vi "main_x.vi"() -> ()   [LabVIEW 2017]
uses:
  <vilib>/Instr/_visa.llb/VISA Configure Serial Port (Instr).vi
panel:
  in  "端口配置":bool
  in  "参数计算":bool
  in  "时漂测试间隔时间(min)":i32=1800000
  in  "时漂测试":bool
  out "时漂":dbl
  out "时漂测试数据":i32[](listbox)
  out "时漂常压输出":string[][](array[string])
  out "错误输出 3":errorcluster caption="错误输出"
  out "Yf.s":dbl[](array[numeric])
  in  "温度显示编号":enum16{""}(ring)
  out "曲线拟合参数":string
  in  "传感器显示编号":enum16{""}(ring)
  out "显示数据":i32[](listbox)
  out "XY图":cluster{dbl[], dbl[]}[](graph)
  out "结束":bool
  out "R5-1":dbl
  out "理论K":dbl
  out "RX":dbl[](array[numeric])
  out "电流":dbl
  out "放大倍数":dbl
  in  "Rx计算":bool
  in  "RsRb计算":bool
  out "Rp":dbl
  out "Rs":dbl
  out "显示数据":string[][](array[string])
  out "数据":string[][](array[string])
  out "错误输出 2":errorcluster caption="错误输出"
  out "压力稳定":bool
  out "压力最小值":dbl
  out "压力最大值":dbl
  out "保存名":string
  out "数据保存路径":path
  out "错误输出":errorcluster
  out "恒温结束时间":string
  out "恒温开始时间":string
  out "恒温结束分钟":i32
  out "恒温结束小时":i32
  out "分钟":i32
  out "小时":i32
  out "开始上电":bool
  out "恒温开始":bool
  out "开始采集":bool
  out "传感器预热":bool
  out "恒温中":bool
  out "温度校验次数":dbl
  out "实时压力kPa":string
  out "实时温度℃":dbl
  out "当前设定温度℃":dbl
  out "温度点":i32
  in  "温度（℃）":dbl[](array[numeric])
  in  "CONST820":refnum<visa-resource-name>="COM3"
  in  "传感器顺序编号（从1开始）":string[](array[string])
  in  "第二路电流 （A）":dbl=1.0
  in  "第二路电压（V）":dbl=5.0
  in  "第一路电压（V）":dbl=5.0
  in  "第一路电流（A）":dbl=1.0
  in  "DH1766-2":refnum<visa-resource-name>="COM5"
  in  "检定次数":i32=1
  in  "恒温时间（分钟）":i32
  in  "传感器预热时间（分钟）":i32
  in  "GWS":refnum<visa-resource-name>="COM4"
  in  "温度上限（℃）":dbl=75.0
  in  "温度下限（℃）":dbl=-45.0
  in  "HP34401":refnum<visa-resource-name>="COM1"
  in  "压力设定值（KPa）":dbl[](array[numeric])
  in  "STOP":bool
  out "loging":string
  out "HP34401A":bool caption="34401A"
  out "GWS":bool
  out "DH1766-2":bool
  out "CONST820":bool
  in  "START":bool
  # "多通道传感器测试系统"
  # "温度设置：如需要进行自动 参数计算，请设置20℃附近常温。如不需要请忽略。\n选择时漂测试 测试完成后会自动进行行程测试。单独点击开始 仅进行行程测试。\n传感器编号从1开始，逐加。\n如需进行时漂测试，请只设置常温常压。"
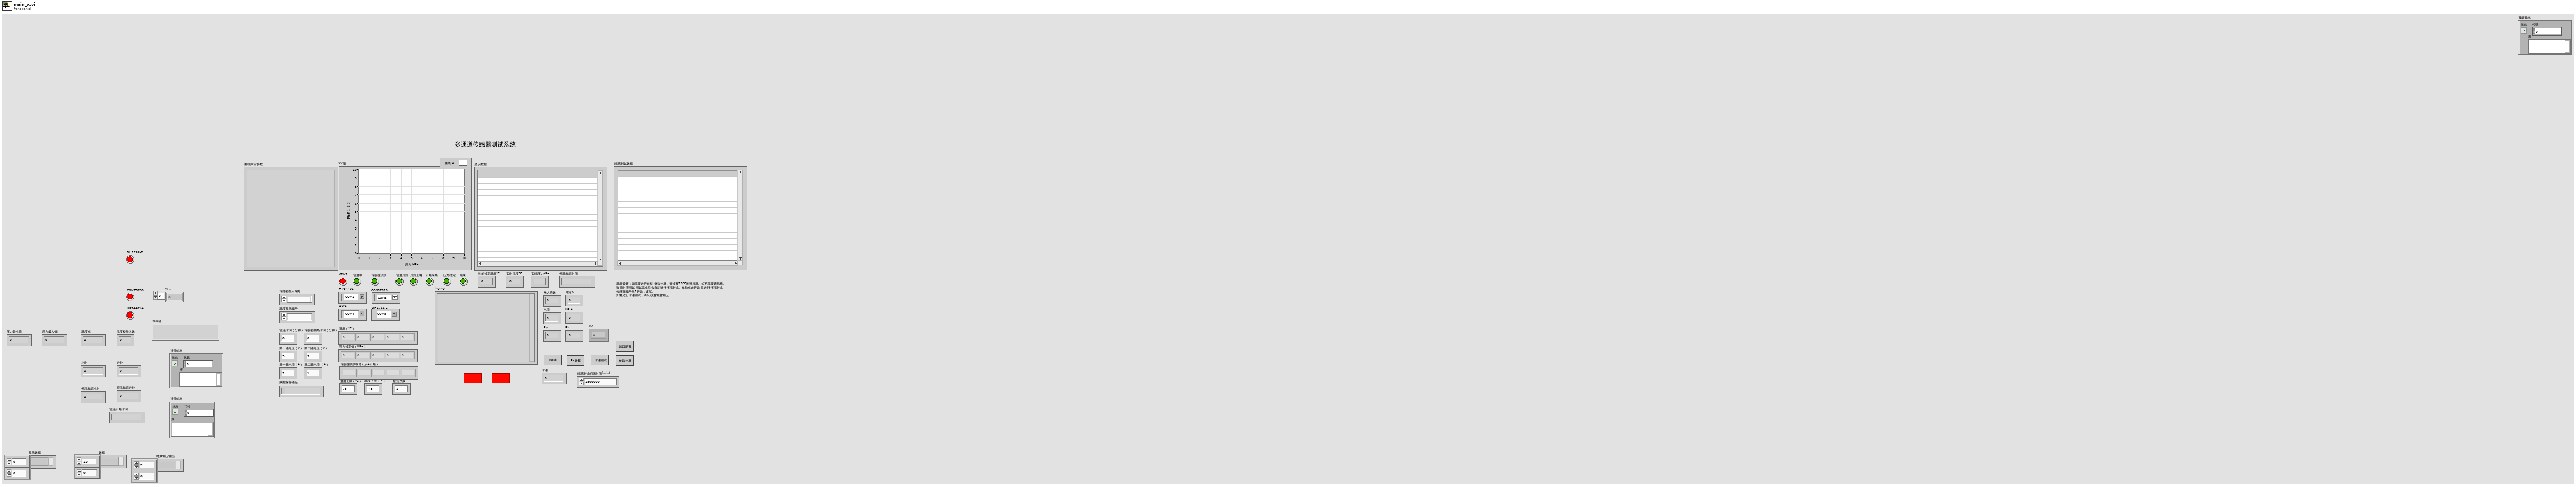
[diagram p1: front panel]
types:
  T1 = enum32{"Invalid", "Standard", "Closed", "Hidden", "Minimized", "Maximized"}
  T2 = enum8{"Enabled", "Disabled", "Disabled and Grayed Out"}
  T3 = enum16{"open", "open or create", "create or replace", "create", "open (read-only)"}
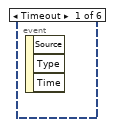
[diagram p2: hidden frame]
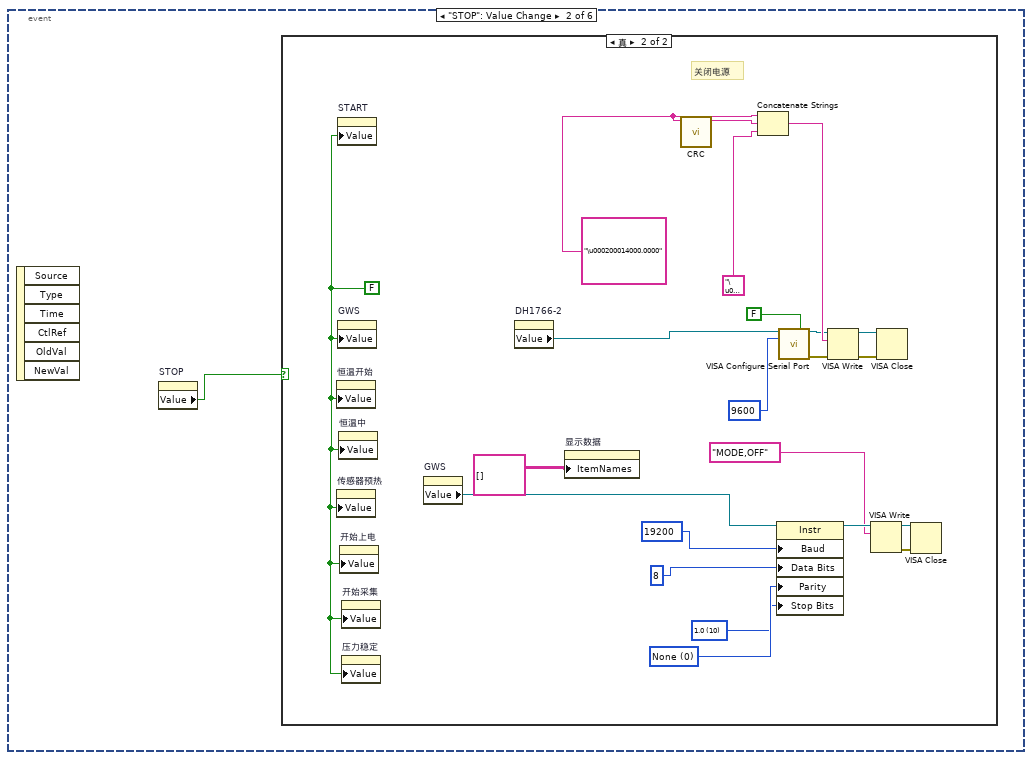
[diagram p3: hidden frame]
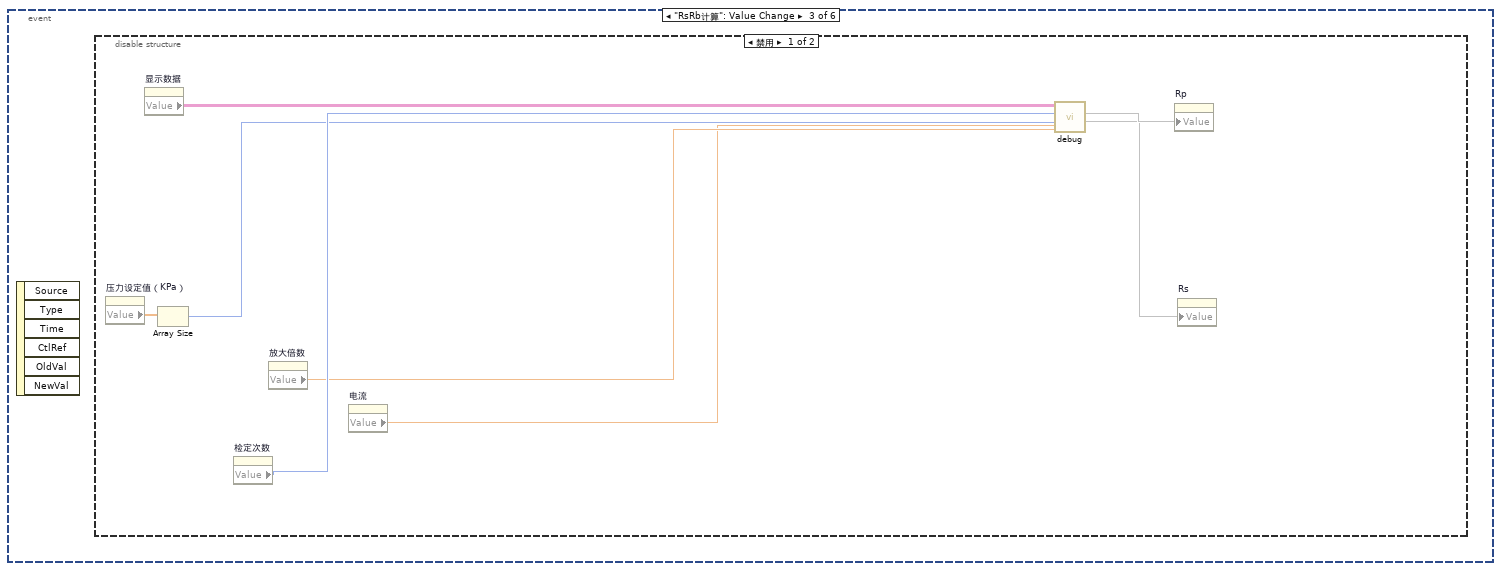
[diagram p5: hidden frame]
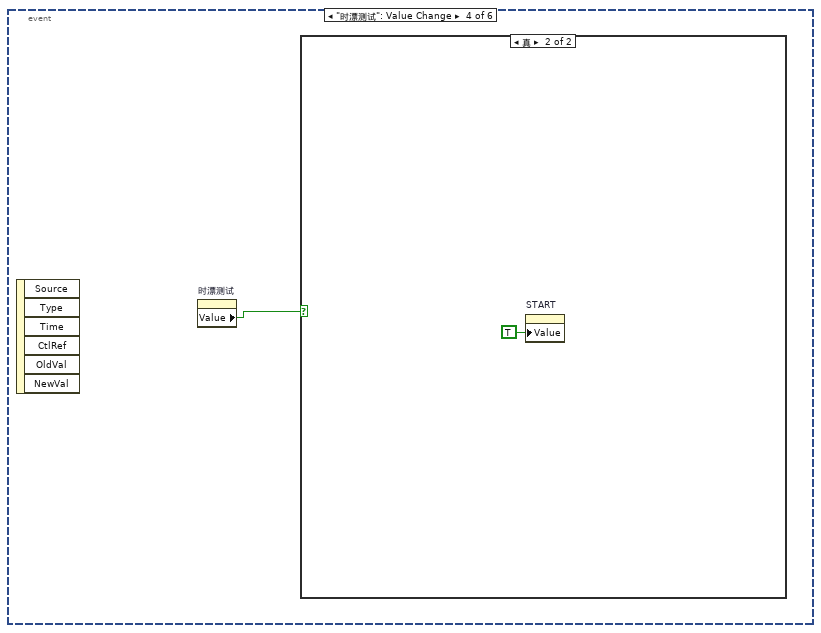
[diagram p7: hidden frame]
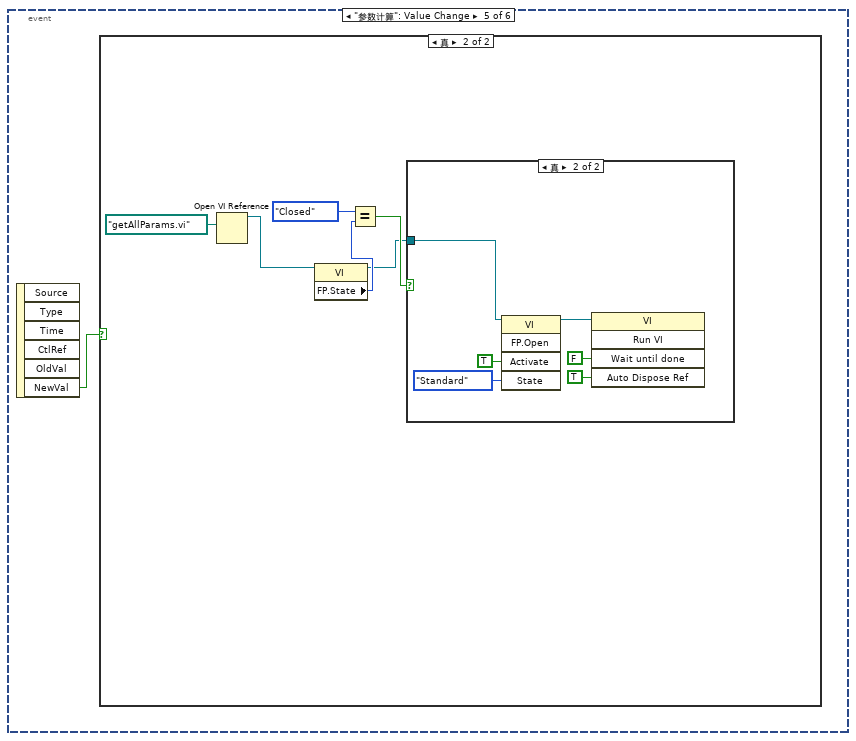
[diagram p9: hidden frame]
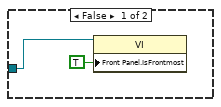
[diagram p11: hidden frame]
diagram:
  n1 = while {
    stop <- FALSE stop-if-true
    n2 = event shown="[5] \"Rx计算\": 值改变" {
      selector: _ -> [_ _ _ _ _ _]
      dyn-events: _ -> [_ _ _ _ _ _]
      timeout: _ -> [_ _ _ _ _ _]
      event Timeout {
        n3 = event-data() -> ()  [unwired: 1 in, 3 out]
      }
      event "STOP": Value Change {
        n4 = event-data() -> ()  [unwired: 1 in, 6 out]
        n5 = property on="STOP" class="Bool (严格)"() -> ("Value"=w2:bool)  [unwired: 2 in, 2 out]
        n6 = case shown="真" w2 {
          frame False {
          }
          frame True {
            w10 = u16 10 items=["1.0"=10, "1.5"=15, "2.0"=20] ("Serial Settings:Stop Bits")
            w11 = u16 0 items=["None", "Odd", "Even", "Mark", "Space"] ("Serial Settings:Parity")
            w9 = "\u000200014000.0000"
            w24 = FALSE ("START")
            # "关闭电源"
            n7 = property on="恒温开始" class="Bool (严格)"("Value"=w24) -> ()  [unwired: 2 in, 2 out]
            n8 = property on="传感器预热" class="Bool (严格)"("Value"=w24) -> ()  [unwired: 2 in, 2 out]
            n9 = property on="START" class="Bool (严格)"("Value"=w24) -> ()  [unwired: 2 in, 2 out]
            n10 = property on="GWS" class="Bool (严格)"("Value"=w24) -> ()  [unwired: 2 in, 2 out]
            n11 = property on="恒温中" class="Bool (严格)"("Value"=w24) -> ()  [unwired: 2 in, 2 out]
            n12 = property on="开始上电" class="Bool (严格)"("Value"=w24) -> ()  [unwired: 2 in, 2 out]
            n13 = property on="开始采集" class="Bool (严格)"("Value"=w24) -> ()  [unwired: 2 in, 2 out]
            n14 = property on="压力稳定" class="Bool (严格)"("Value"=w24) -> ()  [unwired: 2 in, 2 out]
            n15 = property on="GWS" class="VISAName"() -> ("Value"=w5:refnum<visa-resource-name>)  [unwired: 2 in, 2 out]
            n16 = property on="DH1766-2" class="VISAName"() -> ("Value"=w4:refnum<visa-resource-name>)  [unwired: 2 in, 2 out]
            n17 = property on="显示数据" class="MCListbox (严格)"("ItemNames"=string[][] []) -> ()  [unwired: 2 in, 2 out]
            n18 = call "CRC.vi"("命令字符串"=w9) -> ("校验字符串"=w23:string)  [unwired: 10 in]
            n19 = Concatenate Strings(w9, w23, "\u0003" ("字符串")) -> (w20:string)
            n20 = property class="Instr"(reference=w5, "Baud"=u32 19200 ("Serial Settings:Baud Rate"), "Data Bits"=u16 8 ("Serial Settings:Data Bits"), "Parity"=w11, "Stop Bits"=w10) -> (reference out=w17:refnum<visa-resource-name>)  [unwired: 1 in, 1 out]
            n21 = call-poly "VISA Configure Serial Port"("VISA resource name"=w4, "Enable Termination\nChar (T)"=FALSE ("Enable Termination\nChar (T)"), "baud rate (9600)"=u32 9600) -> ("VISA resource name out"=w19:refnum<visa-resource-name>, "error out"=w18:errorcluster)  [unwired: 4 in, 7 out]
            n22 = VISA Write(VISA resource name=w19, write buffer=w20, error in (no error)=w18) -> (VISA resource name out=w22:refnum<visa-resource-name>, error out=w21:errorcluster)  [unwired: 1 out]
            n23 = VISA Write(VISA resource name=w17, write buffer="MODE,OFF" ("写入缓冲区")) -> (VISA resource name out=w15:refnum<visa-resource-name>, error out=w16:errorcluster)  [unwired: 1 in, 1 out]
            n24 = VISA Close(VISA resource name=w22, error in (no error)=w21) -> ()  [unwired: 1 out]
            n25 = VISA Close(VISA resource name=w15, error in (no error)=w16) -> ()  [unwired: 1 out]
          }
        }
      }
      event "RsRb计算": Value Change {
        n26 = event-data() -> ()  [unwired: 1 in, 6 out]
        n27 = disable-structure shown="禁用" {
          frame Disabled {
            n28 = property on="压力设定值（KPa）" class="Arr (严格)"() -> ("Value"=w32:dbl[])  [unwired: 2 in, 2 out]
            n29 = property on="显示数据" class="Arr (严格)"() -> ("Value"=w31:string[][])  [unwired: 2 in, 2 out]
            n30 = Array Size(array=w32) -> (size(s)=w29:i32)
            n31 = property on="检定次数" class="DigNum (严格)"() -> ("Value"=w30:i32)  [unwired: 2 in, 2 out]
            n32 = property on="放大倍数" class="DigNum (严格)"() -> ("Value"=w28:dbl)  [unwired: 2 in, 2 out]
            n33 = property on="电流" class="DigNum (严格)"() -> ("Value"=w27:dbl)  [unwired: 2 in, 2 out]
            n34 = call "debug.vi"("I"=w27, "A"=w28, "压力点个数"=w29, "检定次数"=w30, 11:w31) -> (1:w25, 2:w26)  [unwired: 5 in]
            n35 = property on="Rp" class="DigNum (严格)"("Value"=w26) -> ()  [unwired: 2 in, 2 out]
            n36 = property on="Rs" class="DigNum (严格)"("Value"=w25) -> ()  [unwired: 2 in, 2 out]
          }
          frame Enabled {
          }
        }
      }
      event "时漂测试": Value Change {
        n37 = event-data() -> ()  [unwired: 1 in, 6 out]
        n38 = property on="时漂测试" class="Bool (严格)"() -> ("Value"=w33:bool)  [unwired: 2 in, 2 out]
        n39 = case shown="真" w33 {
          frame False {
          }
          frame True {
            n40 = property on="START" class="Bool (严格)"("Value"=TRUE ("START")) -> ()  [unwired: 2 in, 2 out]
          }
        }
      }
      event "参数计算": Value Change {
        n41 = event-data() -> ("NewVal"=w35:bool)  [unwired: 1 in, 5 out]
        n42 = case shown="真" w35 {
          frame False {
          }
          frame True {
            n43 = Open VI Reference(vi path=path "getAllParams.vi" ("VI路径")) -> (vi reference=w36:refnum<vi>)  [unwired: 5 in, 1 out]
            n44 = property class="VI"(reference=w36) -> (reference out=w37:refnum<vi>, "FP.State"=w40:T1)  [unwired: 1 in, 1 out]
            n45 = Equal?(x=T1."Closed", y=w40) -> (x = y?=w38:bool)
            n46 = case shown="真" w38 {
              tunnel: w37 -> [w42 w44]
              frame False {
                n47 = property class="VI"(reference=w42, "Front Panel.IsFrontmost"=TRUE ("前面板窗口:在最前")) -> ()  [unwired: 1 in, 2 out]
              }
              frame True {
                n48 = invoke class="VI" method="FP.Open"(reference=w44, "Activate"=TRUE ("激活？"), "State"=T1."Standard" ("状态")) -> (reference out=w47:refnum<vi>)  [unwired: 2 in, 4 out]
                n49 = invoke class="VI" method="Run VI"(reference=w47, "Wait until done"=FALSE ("结束前等待"), "Auto Dispose Ref"=TRUE ("自动销毁引用")) -> ()  [unwired: 2 in, 5 out]
              }
            }
          }
        }
      }
      event "Rx计算": Value Change {
        n50 = event-data() -> ()  [unwired: 1 in, 6 out]
        n51 = disable-structure shown="禁用" {
          frame Disabled {
            n52 = property on="压力设定值（KPa）" class="Arr (严格)" props=["Value"]() -> ()  [unwired: 2 in, 3 out]
            n53 = property on="数据" class="Arr (严格)" props=["Value"]() -> ()  [unwired: 2 in, 3 out]
            n54 = property on="压力设定值（KPa）" class="Arr (严格)"() -> ("Value"=w57:dbl[])  [unwired: 2 in, 2 out]
            n55 = Array Size(array=w57) -> (size(s)=w54:i32)
            n56 = property on="数据" class="Arr (严格)"() -> ("Value"=w56:string[][])  [unwired: 2 in, 2 out]
            n57 = property on="检定次数" class="DigNum (严格)"() -> ("Value"=w55:i32)  [unwired: 2 in, 2 out]
            n58 = property on="R5-1" class="DigNum (严格)"() -> ("Value"=w52:dbl)  [unwired: 2 in, 2 out]
            n59 = property on="理论K" class="DigNum (严格)"() -> ("Value"=w51:dbl)  [unwired: 2 in, 2 out]
            n60 = call "getCluster.vi"("数据"=w56, "检定次数"=w55, "压力点个数"=w54, "传感器索引（1开始）"=1, "R5-1"=w52, "理论 K"=w51) -> ("Rx"=w50:dbl[])  [unwired: 2 in, 7 out]
            n61 = property on="RX" class="Arr (严格)"("Value"=w50) -> ()  [unwired: 2 in, 2 out]
          }
          frame Enabled {
          }
        }
      }
    }
  }
  n62 = flat-sequence {
    frame #0 {
      w59 = string[][] []
      w65 = ""
      w66 = 0.0
      w63 = FALSE
      # "时漂测试开始不用规定"
      n63 = disable-structure shown="禁用" {
        frame Disabled {
          n64 = property on="检定次数" class="DigNum (严格)" props=["Value"]() -> ()  [unwired: 3 in, 2 out]
        }
        frame Enabled {
        }
      }
      n65 = property on="START" class="Bool (严格)"("Value"=w63) -> ()  [unwired: 2 in, 2 out]
      n66 = property on="显示数据" class="MCListbox (严格)"("ItemNames"=w59) -> ()  [unwired: 2 in, 2 out]
      n67 = property on="时漂测试数据" class="MCListbox (严格)"("ItemNames"=w59) -> ()  [unwired: 2 in, 2 out]
      n68 = property on="参数计算" class="Bool (严格)"("Value"=FALSE ("参数计算")) -> ()  [unwired: 2 in, 2 out]
      n69 = property on="时漂常压输出" class="Arr (严格)"("Value"=w59) -> ()  [unwired: 2 in, 2 out]
      "GWS" <- w63
      "DH1766-2" <- w63
      "CONST820" <- w63
      "HP34401A" <- w63
      "loging" <- w65
      "温度点" <- 0 ("温度点")
      "当前设定温度℃" <- w66
      "实时温度℃" <- w66
      "实时压力kPa" <- w65
      "温度校验次数" <- 1.0 ("温度校验次数")
      "恒温结束时间" <- "" ("恒温结束时间")
      "数据" <- w59
      "显示数据" <- w59
      "结束" <- w63
      "曲线拟合参数" <- "" ("曲线拟合参数")
      "时漂常压输出" <- w59
    }
    frame #1 {
      n70 = while {
        stop <- FALSE stop-if-true
        # "start循环"
        n71 = property on="START" class="Bool (严格)"() -> ("Value"=w69:bool)  [unwired: 2 in, 2 out]
        n72 = And(x=w69, y=TRUE) -> (x .and. y?=w68:bool)
        n73 = case shown="真" w68 {
          frame False {
          }
          frame True {
            # "start点击判断"
            # "启动系统start"
            n74 = property on="传感器预热时间（分钟）" class="DigNum (严格)"() -> ("Value"=w93:i32)  [unwired: 2 in, 2 out]
            n75 = property on="恒温时间（分钟）" class="DigNum (严格)"() -> ("Value"=w94:i32)  [unwired: 2 in, 2 out]
            n76 = property on="温度下限（℃）" class="DigNum (严格)"() -> ("Value"=w109:dbl)  [unwired: 2 in, 2 out]
            n77 = property on="温度上限（℃）" class="DigNum (严格)"() -> ("Value"=w110:dbl)  [unwired: 2 in, 2 out]
            n78 = property on="GWS" class="VISAName"() -> ("Value"=w122:refnum<visa-resource-name>)  [unwired: 2 in, 2 out]
            n79 = property on="检定次数" class="DigNum (严格)"() -> ("Value"=w91:i32)  [unwired: 2 in, 2 out]
            n80 = property on="DH1766-2" class="VISAName"() -> ("Value"=w120:refnum<visa-resource-name>)  [unwired: 2 in, 2 out]
            n81 = property on="CONST820" class="VISAName"() -> ("Value"=w118:refnum<visa-resource-name>)  [unwired: 2 in, 2 out]
            n82 = property on="HP34401" class="VISAName"() -> ("Value"=w116:refnum<visa-resource-name>)  [unwired: 2 in, 2 out]
            n83 = property on="温度（℃）" class="Arr (严格)"() -> ("Value"=w81:dbl[])  [unwired: 2 in, 2 out]
            n84 = property on="压力设定值（KPa）" class="Arr (严格)"() -> ("Value"=w86:dbl[])  [unwired: 2 in, 2 out]
            n85 = property on="传感器顺序编号（从1开始）" class="Arr (严格)"() -> ("Value"=w76:string[])  [unwired: 2 in, 2 out]
            n86 = Greater Than 0?(x=w91) -> (x > 0?=w90:bool)
            n87 = Greater Than 0?(x=w93) -> (x > 0?=w105:bool)
            n88 = Greater Than 0?(x=w94) -> (x > 0?=w95:bool)
            n89 = Greater Or Equal?(x=w94, y=w93) -> (x >= y?=w92:bool)
            n90 = Array Size(array=w81) -> (size(s)=w80:i32)
            n91 = Array Size(array=w86) -> (size(s)=w84:i32)
            n92 = String Length(string=w122) -> (length=w121:i32)
            n93 = Array Size(array=w76) -> (size(s)=w75:i32)
            n94 = String Length(string=w120) -> (length=w119:i32)
            n95 = String Length(string=w118) -> (length=w117:i32)
            n96 = String Length(string=w116) -> (length=w115:i32)
            n97 = Less Or Equal To 0?(x=w80) -> (x <= 0?=w78:bool)
            n98 = Less Or Equal To 0?(x=w84) -> (x <= 0?=w83:bool)
            n99 = Greater Or Equal?(x=w110, y=w109) -> (x >= y?=w108:bool)
            n100 = Less Or Equal To 0?(x=w75) -> (x <= 0?=w74:bool)
            n101 = Equal?(x=w121, y=0) -> (x = y?=w124:bool)
            n102 = Equal?(x=w119, y=0) -> (x = y?=w123:bool)
            n103 = Equal?(x=w117, y=0) -> (x = y?=w126:bool)
            n104 = Equal?(x=w115, y=0) -> (x = y?=w127:bool)
            n105 = case shown="假" w108 {
              tunnel: ["温度上限>=温度下限 \n" _] -> w102
              frame False {
              }
              frame True {
              }
            }
            n106 = And(x=w95, y=w105) -> (x .and. y?=w89:bool)
            n107 = And(x=w90, y=w89) -> (x .and. y?=w88:bool)
            n108 = And(x=w88, y=w92) -> (x .and. y?=w87:bool)
            n109 = case shown="真" w78 {
              tunnel: [_ "请设置温度\n"] -> w79
              frame False {
              }
              frame True {
              }
            }
            n110 = case shown="真" w83 {
              tunnel: [_ "请设置压力\n"] -> w85
              frame False {
              }
              frame True {
              }
            }
            n111 = case shown="真" w74 {
              tunnel: [_ "请设置传感器编号\n"] -> w71
              frame False {
              }
              frame True {
              }
            }
            n112 = Not(x=w108) -> (.not. x?=w106:bool)
            n113 = Or(x=w123, y=w124) -> (x .or. y?=w125:bool)
            n114 = Or(x=w126, y=w125) -> (x .or. y?=w128:bool)
            n115 = Or(x=w127, y=w128) -> (x .or. y?=w107:bool)
            n116 = case shown="假" w87 {
              tunnel: ["检定次数、恒温时间、传感器预热时间均应大于0、恒温时间>=传感器预热时间 " _] -> w98
              frame False {
              }
              frame True {
              }
            }
            n117 = Not(x=w87) -> (.not. x?=w103:bool)
            n118 = Or(x=w107, y=w106) -> (x .or. y?=w104:bool)
            n119 = case shown="真" w107 {
              tunnel: [_ "部分资源未引用 "] -> w99
              frame False {
              }
              frame True {
              }
            }
            n120 = Or(x=w104, y=w103) -> (x .or. y?=w82:bool)
            n121 = Or(x=w82, y=w83) -> (x .or. y?=w77:bool)
            n122 = Or(x=w77, y=w78) -> (x .or. y?=w73:bool)
            n123 = Or(x=w73, y=w74) -> (x .or. y?=w72:bool)
            n124 = Concatenate Strings(w99, w102, w98, w85, w79, w71) -> (w96:string)
            n125 = Search and Replace String(input string=w96, search string=" " ("搜索字符串"), replace string="\r") -> (result string=w100:string)  [unwired: 5 in, 3 out]
            n126 = case shown="假" w72 {
              tunnel: w100 -> [_ w857]
              frame False {
                # "数值有效判断"
                n127 = property on="时漂测试" class="Bool (严格)"() -> ("Value"=w140:bool)  [unwired: 2 in, 2 out]
                n128 = property on="温度（℃）" class="Arr (严格)"() -> ("Value"=w144:dbl[])  [unwired: 2 in, 2 out]
                n129 = property on="恒温时间（分钟）" class="DigNum (严格)"() -> ("Value"=w136:i32)  [unwired: 2 in, 2 out]
                n130 = property on="时漂测试间隔时间(min)" class="DigNum (严格)"() -> ("Value"=w139:i32)  [unwired: 2 in, 2 out]
                n131 = property on="检定次数" class="DigNum (严格)"("DisabledEnum"=T2."Enabled" ("禁用")) -> ()  [unwired: 2 in, 2 out]
                n132 = property on="结束" class="Bool (严格)"("Value"=FALSE ("结束")) -> ()  [unwired: 2 in, 2 out]
                n133 = Sort 1D Array(array=w144) -> (sorted array=w143:dbl[])
                n134 = Multiply(x=w139, y=8) -> (x*y=w137:i32)
                n135 = Add(x=w137, y=w136) -> (x+y=w135:i32)
                n136 = property on="温度（℃）" class="Arr (严格)"("Value"=w143) -> ()  [unwired: 2 in, 2 out]
                n137 = Number To Decimal String(number=w135) -> (decimal integer string=w134:string)  [unwired: 1 in]
                n138 = case shown="真" w140 {
                  tunnel: w134 -> [_ w147]
                  frame False {
                  }
                  frame True {
                    n139 = Concatenate Strings("计算时间漂移、大约用时：" ("字符串"), w147, " min", "\n") -> (w149:string)
                    n140 = property on="loging" class="Str"("Value"=w149) -> ()  [unwired: 2 in, 2 out]
                  }
                }
                n141 = flat-sequence {
                  frame #0 {
                    # "设置正确"
                    # "启动温箱"
                    n142 = property on="GWS" class="Bool (严格)"() -> ("Value"=w150:bool)  [unwired: 2 in, 2 out]
                    n143 = case shown="假" w150 {
                      frame False {
                        n144 = flat-sequence {
                          tunnel: [w176] -> w156
                          tunnel: [w175] -> w155
                          tunnel: [w199] -> w158
                          tunnel: [w198] -> w157
                          tunnel: w156 -> [w196]
                          tunnel: w155 -> [w195]
                          tunnel: [w215] -> w168
                          tunnel: w158 -> [w215]
                          tunnel: [w214] -> w167
                          tunnel: w157 -> [w214]
                          tunnel: w168 -> [w217]
                          tunnel: w167 -> [w218]
                          tunnel: [w217] -> w166
                          tunnel: [w216] -> w163
                          tunnel: w166 -> [w225]
                          tunnel: [w225] -> w165
                          tunnel: [w224] -> w164
                          tunnel: w163 -> [w224]
                          tunnel: w165 -> [w234]
                          tunnel: w164 -> [w233]
                          tunnel: [w229] -> w161
                          tunnel: [w228] -> w160
                          tunnel: [w238] -> w162
                          tunnel: w161 -> [w238]
                          tunnel: w160 -> [w237]
                          tunnel: [w237] -> w159
                          tunnel: w162 -> [w249]
                          tunnel: w159 -> [w248]
                          tunnel: [w244] -> _
                          frame #0 {
                            w180 = u16 10 items=["1.0"=10, "1.5"=15, "2.0"=20] ("stop bits (10: 1 bit)")
                            n145 = property on="GWS" class="VISAName"() -> ("Value"=w179:refnum<visa-resource-name>)  [unwired: 2 in, 2 out]
                            n146 = property on="loging" class="Str"() -> ("Value"=w172:string)  [unwired: 2 in, 2 out]
                            n147 = Concatenate Strings(w172, "\n启动温箱" ("字符串"), "\n") -> (w171:string)
                            n148 = call-poly "VISA Configure Serial Port"("VISA resource name"=w179, "baud rate (9600)"=u32 19200, "data bits (8)"=u16 8, "parity (0:none)"=enum16{"None", "Odd", "Even", "Mark", "Space"}."None", "stop bits (10: 1 bit)"=w180) -> ("VISA resource name out"=w174:refnum<visa-resource-name>, "error out"=w178:errorcluster)  [unwired: 9 in]
                            n149 = flat-sequence {
                              tunnel: w178 -> [w185]
                              tunnel: [w185] -> w177
                              tunnel: w174 -> [w184]
                              tunnel: [w184] -> w173
                              frame #0 {
                                n150 = Wait (ms)(milliseconds to wait=u32 20 ("等待时间（毫秒）")) -> ()  [unwired: 1 out]
                              }
                            }
                            n151 = property on="loging" class="Str"("Value"=w171) -> ()  [unwired: 2 in, 2 out]
                            n152 = VISA Open(error in (no error)=w177, VISA resource name=w173) -> (VISA resource name=w176:refnum<visa-resource-name>, error out=w175:errorcluster)  [unwired: 3 in]
                          }
                          frame #1 {
                            w203 = i16 1 ("精度(6)")
                            n153 = property on="时漂测试" class="Bool (严格)"() -> ("Value"=w187:bool)  [unwired: 2 in, 2 out]
                            n154 = property on="loging" class="Str"() -> ("Value"=w194:string)  [unwired: 2 in, 2 out]
                            n155 = property on="温度下限（℃）" class="DigNum (严格)"() -> ("Value"=w205:dbl)  [unwired: 2 in, 2 out]
                            n156 = property on="温度上限（℃）" class="DigNum (严格)"() -> ("Value"=w204:dbl)  [unwired: 2 in, 2 out]
                            n157 = case shown="假" w187 {
                              tunnel: [w209 20.0] -> w188
                              frame False {
                                n158 = property on="温度（℃）" class="Arr (严格)"() -> ("Value"=w211:dbl[])  [unwired: 2 in, 2 out]
                                n159 = property on="温度点" class="DigNum (严格)"() -> ("Value"=w210:i32)  [unwired: 2 in, 2 out]
                                n160 = Index Array(array=w211, index=w210) -> (element=w209:dbl)
                                n161 = property on="当前设定温度℃" class="DigNum (严格)"("Value"=w209) -> ()  [unwired: 2 in, 2 out]
                              }
                              frame True {
                              }
                            }
                            n162 = Number To Fractional String(number=w188, precision (6)=i16 2 ("精度(6)")) -> (F-format string=w190:string)  [unwired: 2 in]
                            n163 = Concatenate Strings(w194, "设定温度 " ("字符串"), w190, "\n") -> (w191:string)
                            n164 = Number To Fractional String(number=w188, precision (6)=w203) -> (F-format string=w208:string)  [unwired: 2 in]
                            n165 = Number To Fractional String(number=w204, precision (6)=w203) -> (F-format string=w206:string)  [unwired: 2 in]
                            n166 = Number To Fractional String(number=w205, precision (6)=w203) -> (F-format string=w207:string)  [unwired: 2 in]
                            n167 = property on="loging" class="Str"("Value"=w191) -> ()  [unwired: 2 in, 2 out]
                            n168 = Concatenate Strings("TEMP,S" ("字符串"), w208, " H" ("字符串"), w206, " L" ("字符串"), w207) -> (w197:string)
                            n169 = VISA Write(VISA resource name=w196, write buffer=w197, error in (no error)=w195) -> (VISA resource name out=w199:refnum<visa-resource-name>, error out=w198:errorcluster)  [unwired: 1 out]
                          }
                          frame #2 {
                            n170 = Wait (ms)(milliseconds to wait=u32 100 ("等待时间（毫秒）")) -> ()  [unwired: 1 out]
                          }
                          frame #3 {
                            n171 = Get Date/Time In Seconds() -> (seconds since 1Jan1904=w221:timestamp)
                            n172 = Get Date/Time String(seconds (now)=w221, want seconds? (F)=TRUE ("需要秒？(F)")) -> (time string=w223:string)  [unwired: 1 in, 1 out]
                            n173 = Concatenate Strings("TIME, " ("字符串"), w223) -> (w219:string)
                            n174 = VISA Write(VISA resource name=w217, write buffer=w219, error in (no error)=w218) -> (error out=w216:errorcluster)  [unwired: 2 out]
                          }
                          frame #4 {
                            n175 = Wait (ms)(milliseconds to wait=u32 100 ("等待时间（毫秒）")) -> ()  [unwired: 1 out]
                          }
                          frame #5 {
                            n176 = VISA Write(VISA resource name=w234, write buffer="TEMP？" ("写入缓冲区"), error in (no error)=w233) -> (VISA resource name out=w235:refnum<visa-resource-name>, error out=w230:errorcluster)  [unwired: 1 out]
                            n177 = property class="Instr"(reference=w235, error in=w230) -> (reference out=w232:refnum<visa-resource-name>, error out=w227:errorcluster, "Bytes at Port"=w231:u32)
                            n178 = VISA Read(VISA resource name=w232, byte count=w231, error in (no error)=w227) -> (VISA resource name out=w229:refnum<visa-resource-name>, error out=w228:errorcluster)  [unwired: 2 out]
                          }
                          frame #6 {
                            n179 = Wait (ms)(milliseconds to wait=u32 100 ("等待时间（毫秒）")) -> ()  [unwired: 1 out]
                          }
                          frame #7 {
                            n180 = property on="loging" class="Str"() -> ("Value"=w243:string)  [unwired: 2 in, 2 out]
                            n181 = Concatenate Strings(w243, "温箱已启动" ("字符串"), "\n") -> (w241:string)
                            n182 = property on="GWS" class="Bool (严格)"("Value"=TRUE ("GWS")) -> ()  [unwired: 2 in, 2 out]
                            n183 = VISA Write(VISA resource name=w249, write buffer="MODE,CONSTANT" ("写入缓冲区"), error in (no error)=w248) -> (VISA resource name out=w246:refnum<visa-resource-name>, error out=w245:errorcluster)  [unwired: 1 out]
                            n184 = property on="loging" class="Str"("Value"=w241) -> ()  [unwired: 2 in, 2 out]
                            n185 = VISA Close(VISA resource name=w246, error in (no error)=w245) -> (error out=w244:errorcluster)
                          }
                        }
                      }
                      frame True {
                      }
                    }
                    n186 = disable-structure shown="禁用" {
                      frame Disabled {
                        n187 = property on="loging" class="Str"() -> ("Value"=w153:string)  [unwired: 2 in, 2 out]
                        n188 = Concatenate Strings(w153, "温箱已启动" ("字符串"), "\n") -> (w154:string)
                        n189 = property on="loging" class="Str"("Value"=w154) -> ()  [unwired: 2 in, 2 out]
                      }
                      frame Enabled {
                      }
                    }
                  }
                  frame #1 {
                    # "温箱温度检查"
                    n190 = property on="温度校验次数" class="DigNum (严格)"() -> ("Value"=w252:dbl)  [unwired: 2 in, 2 out]
                    n191 = disable-structure shown="禁用" {
                      frame Disabled {
                        n192 = property on="温度校验次数" class="DigNum (严格)"() -> ("Value"=w254:dbl)  [unwired: 2 in, 2 out]
                        n193 = Greater Than 0?(x=w254) -> (x > 0?=w253:bool)
                        n194 = case shown="真" w253 {
                          frame False {
                          }
                          frame True {
                            n195 = property on="loging" class="Str"() -> ("Value"=w257:string)  [unwired: 2 in, 2 out]
                            n196 = Concatenate Strings(w257, "温箱温度监控" ("字符串"), "\n") -> (w258:string)
                            n197 = property on="loging" class="Str"("Value"=w258) -> ()  [unwired: 2 in, 2 out]
                          }
                        }
                      }
                      frame Enabled {
                      }
                    }
                    n198 = Greater Than 0?(x=w252) -> (x > 0?=w251:bool)
                    n199 = case shown="真" w251 {
                      frame False {
                      }
                      frame True {
                        n200 = while {
                          stop <- w263 stop-if-true
                          n201 = flat-sequence {
                            tunnel: [w270] -> w268
                            tunnel: [w269] -> w267
                            tunnel: [w277] -> w266
                            tunnel: w268 -> [w277]
                            tunnel: [w276] -> w265
                            tunnel: w267 -> [w276]
                            tunnel: w266 -> [w288]
                            tunnel: w265 -> [w287]
                            frame #0 {
                              n202 = property on="GWS" class="VISAName"() -> (error out=w274:errorcluster, "Value"=w275:refnum<visa-resource-name>)  [unwired: 2 in, 1 out]
                              n203 = VISA Flush I/O Buffer(VISA resource name=w275, error in (no error)=w274) -> (VISA resource name out=w272:refnum<visa-resource-name>, error out=w273:errorcluster)  [unwired: 1 in]
                              n204 = VISA Write(VISA resource name=w272, write buffer="TEMP?" ("写入缓冲区"), error in (no error)=w273) -> (VISA resource name out=w270:refnum<visa-resource-name>, error out=w269:errorcluster)  [unwired: 1 out]
                            }
                            frame #1 {
                              n205 = Wait (ms)(milliseconds to wait=u32 100 ("等待时间（毫秒）")) -> ()  [unwired: 1 out]
                            }
                            frame #2 {
                              n206 = property class="Instr"(reference=w288, error in=w287) -> (reference out=w286:refnum<visa-resource-name>, error out=w284:errorcluster, "Bytes at Port"=w285:u32)
                              n207 = VISA Read(VISA resource name=w286, byte count=w285, error in (no error)=w284) -> (read buffer=w279:string)  [unwired: 3 out]
                              n208 = String Subset(string=w279, offset (0)=0 ("偏移量(0)"), length (rest)=5 ("长度（剩余）")) -> (substring=w280:string)
                              n209 = Fract/Exp String To Number(string=w280) -> (number=w283:dbl)  [unwired: 3 in, 1 out]
                              n210 = property on="实时温度℃" class="DigNum (严格)"("Value"=w283) -> ()  [unwired: 2 in, 2 out]
                            }
                            frame #3 {
                              n211 = Wait (ms)(milliseconds to wait=u32 100 ("等待时间（毫秒）")) -> ()  [unwired: 1 out]
                            }
                            frame #4 {
                              w294 = 0.1 ("y")
                              n212 = property on="当前设定温度℃" class="DigNum (严格)"() -> ("Value"=w295:dbl)  [unwired: 2 in, 2 out]
                              n213 = property on="实时温度℃" class="DigNum (严格)"() -> ("Value"=w293:dbl)  [unwired: 2 in, 2 out]
                              n214 = Add(x=w295, y=w294) -> (x+y=w292:dbl)
                              n215 = Subtract(x=w295, y=w294) -> (x-y=w291:dbl)
                              n216 = In Range and Coerce(upper limit=w292, x=w293, lower limit=w291) -> (In Range?=w290:bool)  [unwired: 1 out]
                              n217 = case shown="真" w290 {
                                frame False {
                                }
                                frame True {
                                n218 = property on="温度校验次数" class="DigNum (严格)"() -> ("Value"=w296:dbl)  [unwired: 2 in, 2 out]
                                n219 = Less Or Equal To 0?(x=w296) -> (x <= 0?=w297:bool)
                                n220 = Decrement(x=w296) -> (x-1=w298:dbl)
                                n221 = case shown="真" w297 {
                                frame False {
                                }
                                frame True {
                                n222 = property on="恒温开始" class="Bool (严格)"("Value"=TRUE ("恒温开始")) -> ()  [unwired: 2 in, 2 out]
                                }
                                }
                                n223 = property on="温度校验次数" class="DigNum (严格)"("Value"=w298) -> ()  [unwired: 2 in, 2 out]
                                }
                              }
                            }
                          }
                          n224 = property on="温度校验次数" class="DigNum (严格)"() -> ("Value"=w264:dbl)  [unwired: 2 in, 2 out]
                          n225 = Less Or Equal To 0?(x=w264) -> (x <= 0?=w263:bool)
                        }
                        n226 = property on="loging" class="Str"() -> ("Value"=w262:string)  [unwired: 2 in, 2 out]
                        n227 = Concatenate Strings(w262, "温箱温度监控、恒温检查中" ("字符串"), "\n") -> (w260:string)
                        n228 = property on="loging" class="Str"("Value"=w260) -> ()  [unwired: 2 in, 2 out]
                      }
                    }
                  }
                  frame #2 {
                    # "恒温到达时间计算"
                    n229 = property on="恒温开始" class="Bool (严格)"() -> ("Value"=w300:bool)  [unwired: 2 in, 2 out]
                    n230 = case shown="真" w300 {
                      frame False {
                      }
                      frame True {
                        w310 = TRUE ("恒温中")
                        n231 = Get Date/Time In Seconds() -> (seconds since 1Jan1904=w324:timestamp)
                        n232 = property on="loging" class="Str"() -> ("Value"=w308:string)  [unwired: 2 in, 2 out]
                        n233 = Get Date/Time String(seconds (now)=w324) -> (date string=w303:string, time string=w301:string)  [unwired: 2 in]
                        n234 = property on="恒温中" class="Bool (严格)"("Value"=w310) -> ()  [unwired: 2 in, 2 out]
                        n235 = Concatenate Strings(w308, "开始恒温，计算恒温时间" ("字符串"), "\n") -> (w305:string)
                        n236 = Concatenate Strings(w303, " " ("字符串"), w301) -> (w304:string)
                        n237 = Match Pattern(string=w301, regular expression=":" ("正则表达式")) -> (before substring=w323:string, after substring=w322:string)  [unwired: 1 in, 2 out]
                        n238 = property on="恒温开始时间" class="Str"("Value"=w304) -> ()  [unwired: 2 in, 2 out]
                        n239 = property on="loging" class="Str"("Value"=w305) -> ()  [unwired: 2 in, 2 out]
                        n240 = property on="恒温开始" class="Bool (严格)"("Value"=FALSE ("恒温开始")) -> ()  [unwired: 2 in, 2 out]
                        n241 = property on="传感器预热" class="Bool (严格)"("Value"=w310) -> ()  [unwired: 2 in, 2 out]
                        n242 = Decimal String To Number(string=w323) -> (number=w316:i32)  [unwired: 2 in, 1 out]
                        n243 = Decimal String To Number(string=w322) -> (number=w315:i32)  [unwired: 2 in, 1 out]
                        n244 = property on="分钟" class="DigNum (严格)"("Value"=w315) -> ()  [unwired: 2 in, 2 out]
                        n245 = property on="小时" class="DigNum (严格)"("Value"=w316) -> ()  [unwired: 2 in, 2 out]
                        n246 = property on="恒温时间（分钟）" class="DigNum (严格)"() -> ("Value"=w314:i32)  [unwired: 2 in, 2 out]
                        n247 = call "cal_end_time.vi"("恒温时间"=w314, "分钟"=w315, "小时"=w316) -> ("结束分钟"=w312:i32, "结束小时"=w313:i32)  [unwired: 7 in]
                        n248 = Number To Decimal String(number=w313, width (-)=i16 2 ("宽度(-)")) -> (decimal integer string=w319:string)
                        n249 = Number To Decimal String(number=w312) -> (decimal integer string=w318:string)  [unwired: 1 in]
                        n250 = Concatenate Strings(w319, ":", w318) -> (w311:string)
                        n251 = property on="恒温结束小时" class="DigNum (严格)"("Value"=w313) -> ()  [unwired: 2 in, 2 out]
                        n252 = property on="恒温结束分钟" class="DigNum (严格)"("Value"=w312) -> ()  [unwired: 2 in, 2 out]
                        n253 = property on="恒温结束时间" class="Str"("Value"=w311) -> ()  [unwired: 2 in, 2 out]
                      }
                    }
                  }
                  frame #3 {
                    # "恒温时间到达"
                    n254 = property on="恒温中" class="Bool (严格)"() -> ("Value"=w326:bool)  [unwired: 2 in, 2 out]
                    n255 = property on="传感器预热" class="Bool (严格)"() -> ("Value"=w325:bool)  [unwired: 2 in, 2 out]
                    n256 = disable-structure shown="禁用" {
                      frame Disabled {
                        n257 = property on="loging" class="Str"() -> ("Value"=w329:string)  [unwired: 2 in, 2 out]
                        n258 = Concatenate Strings(w329, "传感器预热" ("字符串"), "\n") -> (w330:string)
                        n259 = property on="loging" class="Str"("Value"=w330) -> ()  [unwired: 2 in, 2 out]
                      }
                      frame Enabled {
                      }
                    }
                    n260 = case shown="真" w326 {
                      frame False {
                      }
                      frame True {
                        n261 = Get Date/Time In Seconds() -> (seconds since 1Jan1904=w361:timestamp)
                        n262 = Get Date/Time String(seconds (now)=w361) -> (time string=w357:string)  [unwired: 2 in, 1 out]
                        n263 = property on="恒温结束分钟" class="DigNum (严格)"() -> ("Value"=w355:i32)  [unwired: 2 in, 2 out]
                        n264 = property on="恒温结束小时" class="DigNum (严格)"() -> ("Value"=w353:i32)  [unwired: 2 in, 2 out]
                        n265 = Match Pattern(string=w357, regular expression=":" ("正则表达式")) -> (before substring=w360:string, after substring=w359:string)  [unwired: 1 in, 2 out]
                        n266 = Decimal String To Number(string=w360) -> (number=w354:i32)  [unwired: 2 in, 1 out]
                        n267 = Decimal String To Number(string=w359) -> (number=w356:i32)  [unwired: 2 in, 1 out]
                        n268 = Equal?(x=w356, y=w355) -> (x = y?=w352:bool)
                        n269 = Equal?(x=w354, y=w353) -> (x = y?=w351:bool)
                        n270 = And(x=w352, y=w351) -> (x .and. y?=w350:bool)
                        n271 = case shown="真" w350 {
                          frame False {
                          }
                          frame True {
                            n272 = property on="loging" class="Str"() -> ("Value"=w366:string)  [unwired: 2 in, 2 out]
                            n273 = property on="开始采集" class="Bool (严格)"("Value"=TRUE ("开始采集")) -> ()  [unwired: 2 in, 2 out]
                            n274 = property on="恒温中" class="Bool (严格)"("Value"=FALSE ("恒温中")) -> ()  [unwired: 2 in, 2 out]
                            n275 = Concatenate Strings(w366, "恒温时间到" ("字符串"), "\n") -> (w363:string)
                            n276 = property on="loging" class="Str"("Value"=w363) -> ()  [unwired: 2 in, 2 out]
                          }
                        }
                      }
                    }
                    n277 = case shown="真" w325 {
                      frame False {
                      }
                      frame True {
                        n278 = property on="恒温时间（分钟）" class="DigNum (严格)"() -> ("Value"=w347:i32)  [unwired: 2 in, 2 out]
                        n279 = property on="传感器预热时间（分钟）" class="DigNum (严格)"() -> ("Value"=w346:i32)  [unwired: 2 in, 2 out]
                        n280 = property on="分钟" class="DigNum (严格)"() -> ("Value"=w344:i32)  [unwired: 2 in, 2 out]
                        n281 = property on="小时" class="DigNum (严格)"() -> ("Value"=w345:i32)  [unwired: 2 in, 2 out]
                        n282 = Get Date/Time In Seconds() -> (seconds since 1Jan1904=w342:timestamp)
                        n283 = Get Date/Time String(seconds (now)=w342) -> (time string=w338:string)  [unwired: 2 in, 1 out]
                        n284 = Subtract(x=w347, y=w346) -> (x-y=w343:i32)
                        n285 = call "cal_end_time.vi"("恒温时间"=w343, "分钟"=w344, "小时"=w345) -> ("结束分钟"=w334:i32, "结束小时"=w336:i32)  [unwired: 7 in]
                        n286 = Match Pattern(string=w338, regular expression=":" ("正则表达式")) -> (before substring=w341:string, after substring=w340:string)  [unwired: 1 in, 2 out]
                        n287 = Decimal String To Number(string=w341) -> (number=w337:i32)  [unwired: 2 in, 1 out]
                        n288 = Decimal String To Number(string=w340) -> (number=w335:i32)  [unwired: 2 in, 1 out]
                        n289 = Equal?(x=w335, y=w334) -> (x = y?=w332:bool)
                        n290 = Equal?(x=w337, y=w336) -> (x = y?=w333:bool)
                        n291 = And(x=w333, y=w332) -> (x .and. y?=w331:bool)
                        n292 = case shown="真" w331 {
                          frame False {
                          }
                          frame True {
                            n293 = property on="传感器预热" class="Bool (严格)"("Value"=FALSE ("传感器预热")) -> ()  [unwired: 2 in, 2 out]
                            n294 = property on="开始上电" class="Bool (严格)"("Value"=TRUE ("开始上电")) -> ()  [unwired: 2 in, 2 out]
                          }
                        }
                      }
                    }
                  }
                  frame #4 {
                    # "开始 设置电源的两路输出端"
                    n295 = property on="开始上电" class="Bool (严格)"() -> ("Value"=w368:bool)  [unwired: 2 in, 2 out]
                    n296 = case shown="真" w368 {
                      frame False {
                      }
                      frame True {
                        n297 = flat-sequence {
                          tunnel: [w378] -> w372
                          tunnel: [w377] -> w370
                          tunnel: w372 -> [w404]
                          tunnel: [w404] -> w371
                          tunnel: w370 -> [w403]
                          tunnel: [w402] -> w369
                          tunnel: w371 -> [w441]
                          tunnel: w369 -> [w440]
                          frame #0 {
                            # "查询设备是否开启的指令"
                            n298 = while {
                              tunnel: [w381] -> w378
                              tunnel: [w380] -> w377
                              stop <- w382 continue-if-true
                              n299 = property on="DH1766-2" class="VISAName"() -> ("Value"=w397:refnum<visa-resource-name>)  [unwired: 2 in, 2 out]
                              n300 = call-poly "VISA Configure Serial Port"("VISA resource name"=w397) -> ("VISA resource name out"=w394:refnum<visa-resource-name>, "error out"=w392:errorcluster)  [unwired: 13 in]
                              n301 = Concatenate Strings("\u000200018\u0004û" ("字符串"), "\u0003" ("字符串")) -> (w393:string)
                              n302 = VISA Write(VISA resource name=w394, write buffer=w393, error in (no error)=w392) -> (VISA resource name out=w391:refnum<visa-resource-name>, error out=w389:errorcluster)  [unwired: 1 out]
                              n303 = flat-sequence {
                                tunnel: w391 -> [w400]
                                tunnel: [w400] -> w390
                                tunnel: w389 -> [w399]
                                tunnel: [w399] -> w388
                                frame #0 {
                                n304 = Wait (ms)(milliseconds to wait=u32 100 ("等待时间（毫秒）")) -> ()  [unwired: 1 out]
                                }
                              }
                              n305 = property class="Instr"(reference=w390, error in=w388) -> (reference out=w385:refnum<visa-resource-name>, error out=w387:errorcluster, "Bytes at Port"=w386:u32)
                              n306 = VISA Read(VISA resource name=w385, byte count=w386, error in (no error)=w387) -> (VISA resource name out=w381:refnum<visa-resource-name>, read buffer=w384:string, error out=w380:errorcluster)  [unwired: 1 out]
                              n307 = Wait Until Next ms Multiple(millisecond multiple=u32 10 ("毫秒倍数")) -> ()  [unwired: 1 out]
                              n308 = Equal?(x=w384, y="") -> (x = y?=w382:bool)
                              n309 = case shown="真" w382 {
                                frame False {
                                }
                                frame True {
                                n310 = One Button Dialog(message="DH1766电源未开启" ("消息")) -> ()  [unwired: 1 in, 1 out]
                                }
                              }
                            }
                            n311 = property on="loging" class="Str"() -> ("Value"=w376:string)  [unwired: 2 in, 2 out]
                            n312 = Concatenate Strings(w376, "电源输出，开始上电，预热传感器" ("字符串"), "\n") -> (w373:string)
                            n313 = property on="loging" class="Str"("Value"=w373) -> ()  [unwired: 2 in, 2 out]
                          }
                          frame #1 {
                            # "顺序指令执行"
                            n314 = property on="第一路电流（A）" class="DigNum (严格)"() -> ("Value"=w411:dbl)  [unwired: 2 in, 2 out]
                            n315 = property on="第一路电压（V）" class="DigNum (严格)"() -> ("Value"=w410:dbl)  [unwired: 2 in, 2 out]
                            n316 = property on="第二路电压（V）" class="DigNum (严格)"() -> ("Value"=w408:dbl)  [unwired: 2 in, 2 out]
                            n317 = property on="第二路电流 （A）" class="DigNum (严格)"() -> ("Value"=w409:dbl)  [unwired: 2 in, 2 out]
                            n318 = Build Array(w411, w410, w409, w408) -> (w406:dbl[])
                            n319 = Array Size(array=w406) -> (size(s)=w407:i32)
                            n320 = Build Array("\u0002000000", "\u0002000010", "\u0002010000", "\u0002010010") -> (w405:string[])
                            n321 = for {
                              N: w407 -> [_]
                              tunnel: w406 -> [w420] mode=indexing
                              tunnel: w405 -> [w419] mode=indexing
                              tunnel: w404 -> [w418]
                              shift-right: [w416] -> w402
                              shift-left: w403 -> [w417]
                              n322 = flat-sequence {
                                tunnel: w420 -> [w425]
                                tunnel: w419 -> [w424]
                                tunnel: w418 -> [w423]
                                tunnel: w417 -> [w422]
                                tunnel: [w421] -> w416
                                frame #0 {
                                n323 = Number To Fractional String(number=w425, width (-)=7, precision (6)=i16 4 ("精度(6)")) -> (F-format string=w434:string)  [unwired: 1 in]
                                n324 = Search and Replace String(input string=w434, search string=" " ("搜索字符串"), replace string="0" ("子字符串(\"\")"), offset=0 ("偏移量(0)")) -> (result string=w435:string)  [unwired: 4 in, 3 out]
                                n325 = Concatenate Strings(w424, w435) -> (w429:string)
                                n326 = call "CRC.vi"("命令字符串"=w429) -> ("校验字符串"=w428:string)  [unwired: 10 in]
                                n327 = Concatenate Strings(w429, w428, "\u0003" ("字符串")) -> (w427:string)
                                n328 = VISA Write(VISA resource name=w423, write buffer=w427, error in (no error)=w422) -> (error out=w421:errorcluster)  [unwired: 2 out]
                                }
                                frame #1 {
                                n329 = Wait (ms)(milliseconds to wait=u32 100 ("等待时间（毫秒）")) -> ()  [unwired: 1 out]
                                }
                              }
                            }
                          }
                          frame #2 {
                            w444 = "\u000200014111.0000"
                            # "结束配置"
                            n330 = property on="开始上电" class="Bool (严格)"("Value"=FALSE ("开始上电")) -> ()  [unwired: 2 in, 2 out]
                            n331 = call "CRC.vi"("命令字符串"=w444) -> ("校验字符串"=w445:string)  [unwired: 10 in]
                            n332 = Concatenate Strings(w444, w445, "\u0003" ("字符串")) -> (w446:string)
                            n333 = VISA Write(VISA resource name=w441, write buffer=w446, error in (no error)=w440) -> (VISA resource name out=w443:refnum<visa-resource-name>, error out=w442:errorcluster)  [unwired: 1 out]
                            n334 = VISA Close(VISA resource name=w443, error in (no error)=w442) -> (error out=→"错误输出":errorcluster)
                          }
                        }
                      }
                    }
                  }
                  frame #5 {
                    # "开始采集数据"
                    n335 = property on="开始采集" class="Bool (严格)"() -> ("Value"=w448:bool)  [unwired: 2 in, 2 out]
                    n336 = case shown="真" w448 {
                      frame False {
                      }
                      frame True {
                        n337 = property on="时漂测试" class="Bool (严格)"() -> ("Value"=w453:bool)  [unwired: 2 in, 2 out]
                        n338 = Get Date/Time String() -> (date string=w472:string, time string=w459:string)  [unwired: 3 in]
                        n339 = Search and Replace String(input string=w472, search string="/" ("搜索字符串"), replace string="" ("替换字符串(\"\")")) -> (result string=w479:string)  [unwired: 5 in, 3 out]
                        n340 = Search and Replace String(input string=w459, search string=":" ("搜索字符串"), replace string="" ("替换字符串(\"\")")) -> (result string=w463:string)  [unwired: 5 in, 3 out]
                        n341 = property on="loging" class="Str"() -> ("Value"=w469:string)  [unwired: 2 in, 2 out]
                        n342 = Search and Replace String(input string=w479, search string="/" ("搜索字符串"), replace string="" ("替换字符串(\"\")")) -> (result string=w476:string)  [unwired: 5 in, 3 out]
                        n343 = Concatenate Strings(w469, "恒温变压数据采集中" ("字符串"), "\n") -> (w466:string)
                        n344 = Search and Replace String(input string=w463, search string=":" ("搜索字符串"), replace string="" ("替换字符串(\"\")")) -> (result string=w458:string)  [unwired: 5 in, 3 out]
                        n345 = Concatenate Strings(w476, "" ("字符串")) -> (w474:string)
                        n346 = property on="loging" class="Str"("Value"=w466) -> ()  [unwired: 2 in, 2 out]
                        n347 = Concatenate Strings(w474, "_" ("字符串"), w458) -> (w455:string)
                        "保存名" <- w455
                        n348 = property on="当前设定温度℃" class="DigNum (严格)"() -> ("Value"=w470:dbl)  [unwired: 2 in, 2 out]
                        n349 = Number To Fractional String(number=w470, precision (6)=i16 1 ("精度(6)")) -> (F-format string=w452:string)  [unwired: 2 in]
                        n350 = Search and Replace String(input string=w452, search string="." ("搜索字符串"), replace string="" ("替换字符串(\"\")")) -> (result string=w449:string)  [unwired: 5 in, 3 out]
                        n351 = Concatenate Strings(w455, "_" ("字符串"), w449) -> (w473:string)
                        n352 = String To Path(string=w473) -> (path=→"数据保存路径":path)
                        n353 = case shown="真" w453 {
                          frame False {
                          }
                          frame True {
                            # "时漂执行序列"
                            # "时间漂移测试"
                            n354 = flat-sequence {
                              frame #0 {
                                n355 = for {
                                N: 9 -> [_]
                                i -> [w643]
                                # "执行序列"
                                n356 = flat-sequence {
                                tunnel: [w659] -> w654
                                tunnel: [w658] -> w648
                                tunnel: [w656] -> w644
                                tunnel: [w663] -> w655
                                tunnel: w654 -> [w663]
                                tunnel: [w662] -> w653
                                tunnel: w648 -> [w662]
                                tunnel: [w660] -> w645
                                tunnel: w644 -> [w660]
                                tunnel: w655 -> [w669]
                                tunnel: w653 -> [w668]
                                tunnel: [w667] -> w652
                                tunnel: [w666] -> w651
                                tunnel: [w665] -> w647
                                tunnel: [w664] -> w646
                                tunnel: w645 -> [w664]
                                tunnel: w652 -> [w683]
                                tunnel: w651 -> [w682]
                                tunnel: [w681] -> w650
                                tunnel: [w680] -> w649
                                tunnel: w647 -> [w679]
                                tunnel: w646 -> [w678]
                                tunnel: w650 -> [w707]
                                tunnel: w649 -> [w706]
                                tunnel: w643 -> [w753]
                                frame #0 {
                                w656 = 100.0 ("设定")
                                # "压力固定值"
                                n357 = property on="CONST820" class="VISAName"() -> ("Value"=w657:refnum<visa-resource-name>)  [unwired: 2 in, 2 out]
                                n358 = call "设定压力.vi"("设定"=w656, "VISA resource name"=w657) -> ("错误输出"=w658:errorcluster, "VISA资源名称输出"=w659:refnum<visa-resource-name>)  [unwired: 1 in]
                                }
                                frame #1 {
                                n359 = Wait (ms)(milliseconds to wait=u32 100 ("毫秒计时值")) -> ()  [unwired: 1 out]
                                }
                                frame #2 {
                                n360 = while {
                                tunnel: w669 -> [w674]
                                tunnel: w668 -> [w673]
                                tunnel: [w676] -> w665
                                tunnel: [w672] -> w667
                                tunnel: [w671] -> w666
                                stop <- w676 stop-if-true
                                # "1稳定 0不稳定"
                                n361 = call "压力稳定状态.vi"("error in (no error) 2"=w673, "VISA resource name"=w674) -> ("错误输出"=w671:errorcluster, "状态(1稳定)"=w670:string, "VISA资源名称输出"=w672:refnum<visa-resource-name>)  [unwired: 1 in]
                                n362 = Wait Until Next ms Multiple(millisecond multiple=u32 10 ("毫秒倍数")) -> ()  [unwired: 1 out]
                                n363 = Decimal String To Number(string=w670) -> (number=w677:i32)  [unwired: 2 in, 1 out]
                                n364 = Greater Than 0?(x=w677) -> (x > 0?=w676:bool)
                                }
                                n365 = property on="压力稳定" class="Bool (严格)"("Value"=w665) -> ()  [unwired: 2 in, 2 out]
                                }
                                frame #3 {
                                n366 = case shown="真" w679 {
                                tunnel: w683 -> [w685 w690]
                                tunnel: w682 -> [w684 w689]
                                tunnel: [w685 w688] -> w681
                                tunnel: [w684 w687] -> w680
                                tunnel: w678 -> [_ w686]
                                frame False {
                                }
                                frame True {
                                n367 = while {
                                tunnel: w690 -> [w696]
                                tunnel: w689 -> [w697]
                                tunnel: [w695] -> w688
                                tunnel: [w693] -> w687
                                tunnel: [w692] -> _
                                tunnel: w686 -> [w691]
                                stop <- w699 stop-if-true
                                n368 = call "CONST820目标压力测量.vi"("error in (no error) 2"=w697, "VISA resource name"=w696) -> ("错误输出"=w693:errorcluster, "目标压力值"=w694:string, "VISA资源名称输出"=w695:refnum<visa-resource-name>)  [unwired: 1 in]
                                n369 = Wait Until Next ms Multiple(millisecond multiple=u32 10 ("毫秒倍数")) -> ()  [unwired: 1 out]
                                n370 = Match Pattern(string=w694, regular expression="," ("正则表达式")) -> (before substring=w692:string)  [unwired: 1 in, 3 out]
                                n371 = property on="实时压力kPa" class="Str"("Value"=w692) -> ()  [unwired: 2 in, 2 out]
                                n372 = Fract/Exp String To Number(string=w692) -> (number=w703:dbl)  [unwired: 3 in, 1 out]
                                n373 = Divide(x=w703, y=w691) -> (x/y=w702:dbl)
                                n374 = In Range and Coerce(upper limit=1.0005 ("上限"), x=w702, lower limit=0.9995 ("下限")) -> (In Range?=w699:bool)  [unwired: 1 out]
                                }
                                }
                                }
                                }
                                frame #4 {
                                n375 = VISA Close(VISA resource name=w707, error in (no error)=w706) -> (error out=→"错误输出 3":errorcluster)
                                }
                                frame #5 {
                                # "可视化"
                                # "数据采集"
                                n376 = property on="当前设定温度℃" class="DigNum (严格)"() -> ("Value"=w711:dbl)  [unwired: 2 in, 2 out]
                                n377 = property on="GWS" class="VISAName"() -> (error out=w710:errorcluster, "Value"=w709:refnum<visa-resource-name>)  [unwired: 2 in, 1 out]
                                n378 = while {
                                tunnel: w709 -> [w717]
                                tunnel: w710 -> [w716]
                                tunnel: w711 -> [w715]
                                tunnel: [w714] -> w708
                                tunnel: [w713] -> w712
                                stop <- w714 stop-if-true
                                w718 = 0.1
                                # "再次判断温度设置"
                                n379 = call "get_temp.vi"("错误输入（无错误）"=w716, "VISA资源名称"=w717) -> ("实时温度"=w713:dbl)  [unwired: 7 in, 2 out]
                                n380 = property on="实时温度℃" class="DigNum (严格)"("Value"=w713) -> ()  [unwired: 2 in, 2 out]
                                n381 = Add(x=w715, y=w718) -> (x+y=w719:dbl)
                                n382 = Subtract(x=w715, y=w718) -> (x-y=w720:dbl)
                                n383 = In Range and Coerce(upper limit=w719, x=w713, lower limit=w720) -> (In Range?=w714:bool)  [unwired: 1 out]
                                }
                                n384 = case shown="真" w708 {
                                tunnel: w712 -> [_ w724]
                                frame False {
                                }
                                frame True {
                                w727 = u16 0 items=["DC Voltage", "AC Voltage", "2 - Wire Resistance", "4 - Wire Resistance", "DC Current", "AC Current", "Frequency", "Period", "Continuity", "Diode Checking", "VDC:VDC Ratio", "Temperature", "Capacitance"] ("Function (0: DC Voltage)")
                                w734 = ""
                                n385 = property on="传感器顺序编号（从1开始）" class="Arr (严格)"() -> ("Value"=w723:string[])  [unwired: 2 in, 2 out]
                                n386 = property on="HP34401" class="VISAName"() -> ("Value"=w722:refnum<visa-resource-name>)  [unwired: 2 in, 2 out]
                                n387 = Get Date/Time String(want seconds? (F)=TRUE ("disable buffering (T)")) -> (time string=w745:string)  [unwired: 2 in, 1 out]
                                n388 = property on="实时压力kPa" class="Str"() -> ("Value"=w743:string)  [unwired: 2 in, 2 out]
                                n389 = Number To Fractional String(number=w724) -> (F-format string=w744:string)  [unwired: 3 in]
                                n390 = Array Size(array=w723) -> (size(s)=w742:i32)
                                n391 = Interleave 1D Arrays(w723, string[] [" ", " ", " ", " ", " "]) -> (w735:string[])
                                n392 = Multiply(x=2, y=w742) -> (x*y=w726:i32)
                                n393 = for {
                                N: w726 -> [_]
                                tunnel: w722 -> [w750]
                                tunnel: w727 -> [w749]
                                tunnel: [w747] -> w725 mode=indexing
                                n394 = call "Agilent 34401.vi"("Function (0: DC Voltage)"=w749, "VISA resource name"=w750) -> ("Measurement"=w748:dbl)  [unwired: 1 in, 1 out]
                                n395 = Number To Fractional String(number=w748) -> (F-format string=w747:string)  [unwired: 3 in]
                                }
                                n396 = Add(x=3, y=w726) -> (x+y=w737:i32)
                                n397 = Build Array (concatenate)(w745, w744, w743, w725) -> (w730:string[])
                                n398 = Build Array (concatenate)(w734, w734, w734, w735) -> (w732:string[])
                                n399 = property on="时漂常压输出" class="Arr (严格)"() -> ("Value"=w731:string[][])  [unwired: 2 in, 2 out]
                                n400 = Array Subset(array=string[] ["时间", "温度（℃）", "压力（KPa）", "电压1（V）", "桥压1（V）", "电压2（V）", "桥压2（V）", "电压3（V）", "桥压3（V）", "电压4（V）", "桥压4（V）", "电压5（V）", "桥压5（V）"], index=0 ("索引"), length=w737) -> (w733:string[])
                                n401 = Build Array (concatenate)(w731, w730) -> (w728:string[][])
                                n402 = Build Array(w733, w732) -> (w729:string[][])
                                n403 = Insert Into Array(array=w729, new element=w728) -> (w721:string[][])  [unwired: 2 in]
                                n404 = property on="时漂常压输出" class="Arr (严格)"("Value"=w728) -> ()  [unwired: 2 in, 2 out]
                                n405 = property on="时漂测试数据" class="MCListbox (严格)"("ItemNames"=w721) -> ()  [unwired: 2 in, 2 out]
                                }
                                }
                                }
                                frame #6 {
                                n406 = property on="压力稳定" class="Bool (严格)"("Value"=FALSE ("压力稳定")) -> ()  [unwired: 2 in, 2 out]
                                }
                                frame #7 {
                                n407 = Less?(x=w753, y=8.0) -> (x < y?=w752:bool)
                                n408 = case shown="真" w752 {
                                frame False {
                                }
                                frame True {
                                n409 = property on="时漂测试间隔时间(min)" class="DigNum (严格)"() -> ("Value"=w757:i32)  [unwired: 2 in, 2 out]
                                n410 = Multiply(x=w757, y=60000) -> (x*y=w755:i32)
                                n411 = Wait Until Next ms Multiple(millisecond multiple=w755) -> ()  [unwired: 1 out]
                                }
                                }
                                }
                                }
                                }
                              }
                              frame #1 {
                                n412 = property on="开始采集" class="Bool (严格)"("Value"=FALSE ("开始采集")) -> ()  [unwired: 2 in, 2 out]
                                n413 = property on="压力稳定" class="Bool (严格)"("Value"=FALSE ("压力稳定")) -> ()  [unwired: 2 in, 2 out]
                                n414 = property on="结束" class="Bool (严格)"("Value"=TRUE ("结束")) -> ()  [unwired: 2 in, 2 out]
                              }
                            }
                          }
                        }
                        n415 = Not(x=w453) -> (.not. x?=w454:bool)
                        n416 = case shown="真" w454 {
                          frame False {
                          }
                          frame True {
                            # "不是时漂执行该序列"
                            n417 = property on="压力设定值（KPa）" class="Arr (严格)"() -> ("Value"=w490:dbl[])  [unwired: 2 in, 2 out]
                            n418 = property on="压力设定值（KPa）" class="Arr (严格)"() -> ("Value"=w496:dbl[])  [unwired: 2 in, 2 out]
                            n419 = Reverse 1D Array(array=w490) -> (reversed array=w492:dbl[])
                            n420 = Array Max & Min(array=w490) -> (max value=w487:dbl, min value=w488:dbl)  [unwired: 2 out]
                            n421 = property on="检定次数" class="DigNum (严格)"() -> ("Value"=w498:i32)  [unwired: 2 in, 2 out]
                            n422 = Sort 1D Array(array=w496) -> (sorted array=w495:dbl[])
                            n423 = Multiply(x=1.01, y=w487) -> (x*y=w491:dbl)
                            n424 = Multiply(x=w488, y=0.99) -> (x*y=w489:dbl)
                            n425 = property on="压力设定值（KPa）" class="Arr (严格)"("Value"=w495) -> ()  [unwired: 2 in, 2 out]
                            n426 = Array Size(array=w495) -> (size(s)=w501:i32)
                            n427 = Increment(x=w501) -> (x+1=w500:i32)
                            n428 = Build Array (concatenate)(w489, w490, w491, w492) -> (w483:dbl[])
                            n429 = Array Max & Min(array=w483) -> (max value=→"压力最大值":dbl, min value=→"压力最小值":dbl)  [unwired: 2 out]
                            n430 = Multiply(x=2, y=w500) -> (x*y=w497:i32)
                            n431 = Multiply(x=w497, y=w498) -> (x*y=w482:i32)
                            n432 = Array Size(array=w483) -> (size(s)=w484:i32)
                            n433 = flat-sequence {
                              tunnel: w483 -> [w504]
                              tunnel: w484 -> [w503]
                              tunnel: w482 -> [w502]
                              frame #0 {
                                n434 = for {
                                N: w502 -> [_]
                                tunnel: w504 -> [w522]
                                tunnel: w503 -> [w507]
                                i -> [w520]
                                # "执行序列"
                                n435 = Greater Or Equal?(x=w520, y=w507) -> (x >= y?=w521:bool)
                                n436 = case shown="真" w521 {
                                tunnel: w520 -> [w523 w526]
                                tunnel: w507 -> [_ w525]
                                tunnel: [w523 w524] -> w519
                                frame False {
                                }
                                frame True {
                                n437 = Quotient & Remainder(x=w526, y=w525) -> (x-y*floor(x/y)=w524:i32)  [unwired: 1 out]
                                }
                                }
                                n438 = Index Array(array=w522, index=w519) -> (element=w505:dbl)
                                n439 = flat-sequence {
                                tunnel: w505 -> [w529]
                                tunnel: [w528] -> w517
                                tunnel: [w527] -> w506
                                tunnel: [w533] -> w518
                                tunnel: w517 -> [w533]
                                tunnel: [w532] -> w516
                                tunnel: w506 -> [w532]
                                tunnel: w518 -> [w545]
                                tunnel: w516 -> [w544]
                                tunnel: [w542] -> w515
                                tunnel: [w541] -> w514
                                tunnel: [w540] -> w513
                                tunnel: w505 -> [w535]
                                tunnel: w515 -> [w554]
                                tunnel: w514 -> [w560]
                                tunnel: w513 -> [w559]
                                tunnel: w505 -> [w558]
                                tunnel: [w557] -> w512
                                tunnel: [w556] -> w511
                                tunnel: [w555] -> w510
                                tunnel: [w554] -> w508
                                tunnel: w512 -> [_]
                                tunnel: w511 -> [w592]
                                tunnel: w510 -> [w591]
                                tunnel: [w589] -> w509
                                tunnel: w508 -> [w589]
                                tunnel: w509 -> [w595]
                                frame #0 {
                                n440 = property on="CONST820" class="VISAName"() -> ("Value"=w530:refnum<visa-resource-name>)  [unwired: 2 in, 2 out]
                                n441 = call "设定压力.vi"("设定"=w529, "VISA resource name"=w530) -> ("错误输出"=w527:errorcluster, "VISA资源名称输出"=w528:refnum<visa-resource-name>)  [unwired: 1 in]
                                }
                                frame #1 {
                                n442 = Wait (ms)(milliseconds to wait=u32 100 ("毫秒计时值")) -> ()  [unwired: 1 out]
                                }
                                frame #2 {
                                n443 = property on="压力最大值" class="DigNum (严格)"() -> ("Value"=w536:dbl)  [unwired: 2 in, 2 out]
                                n444 = property on="压力最小值" class="DigNum (严格)"() -> ("Value"=w537:dbl)  [unwired: 2 in, 2 out]
                                n445 = while {
                                tunnel: w545 -> [w550]
                                tunnel: w544 -> [w549]
                                tunnel: [w552] -> w543
                                tunnel: [w548] -> w541
                                tunnel: [w547] -> w540
                                stop <- w552 stop-if-true
                                # "1稳定 0不稳定"
                                n446 = call "压力稳定状态.vi"("error in (no error) 2"=w549, "VISA resource name"=w550) -> ("错误输出"=w547:errorcluster, "状态(1稳定)"=w546:string, "VISA资源名称输出"=w548:refnum<visa-resource-name>)  [unwired: 1 in]
                                n447 = Wait Until Next ms Multiple(millisecond multiple=u32 10 ("毫秒倍数")) -> ()  [unwired: 1 out]
                                n448 = Decimal String To Number(string=w546) -> (number=w553:i32)  [unwired: 2 in, 1 out]
                                n449 = Greater Than 0?(x=w553) -> (x > 0?=w552:bool)
                                }
                                n450 = Equal?(x=w535, y=w536) -> (x = y?=w539:bool)
                                n451 = Equal?(x=w537, y=w535) -> (x = y?=w538:bool)
                                n452 = Not Or(1:w539, 2:w538) -> (0:w534:bool)
                                n453 = And(x=w534, y=w543) -> (x .and. y?=w542:bool)
                                n454 = property on="压力稳定" class="Bool (严格)"("Value"=w542) -> ()  [unwired: 2 in, 2 out]
                                }
                                frame #3 {
                                n455 = case shown="真" w554 {
                                tunnel: w560 -> [w562 w574]
                                tunnel: w559 -> [w561 w573]
                                tunnel: [w563 w572] -> w557
                                tunnel: w558 -> [w565 w571]
                                tunnel: [w562 w570] -> w556
                                tunnel: [w561 w569] -> w555
                                frame False {
                                n456 = property on="压力最小值" class="DigNum (严格)"() -> ("Value"=w566:dbl)  [unwired: 2 in, 2 out]
                                n457 = Equal?(x=w566, y=w565) -> (x = y?=w564:bool)
                                n458 = case shown="真" w564 {
                                tunnel: ["反行程" "正行程"] -> w563
                                frame False {
                                }
                                frame True {
                                }
                                }
                                }
                                frame True {
                                n459 = while {
                                tunnel: w574 -> [w578]
                                tunnel: w573 -> [w579]
                                tunnel: [w577] -> w570
                                tunnel: [w575] -> w569
                                tunnel: [w587] -> w572
                                tunnel: w571 -> [w585]
                                stop <- w581 stop-if-true
                                n460 = call "CONST820目标压力测量.vi"("error in (no error) 2"=w579, "VISA resource name"=w578) -> ("错误输出"=w575:errorcluster, "目标压力值"=w576:string, "VISA资源名称输出"=w577:refnum<visa-resource-name>)  [unwired: 1 in]
                                n461 = Wait Until Next ms Multiple(millisecond multiple=u32 10 ("毫秒倍数")) -> ()  [unwired: 1 out]
                                n462 = Match Pattern(string=w576, regular expression="," ("正则表达式")) -> (before substring=w587:string)  [unwired: 1 in, 3 out]
                                n463 = property on="实时压力kPa" class="Str"("Value"=w587) -> ()  [unwired: 2 in, 2 out]
                                n464 = Fract/Exp String To Number(string=w587) -> (number=w586:dbl)  [unwired: 3 in, 1 out]
                                n465 = Divide(x=w586, y=w585) -> (x/y=w584:dbl)
                                n466 = In Range and Coerce(upper limit=1.0005 ("上限"), x=w584, lower limit=0.9995 ("下限")) -> (In Range?=w581:bool)  [unwired: 1 out]
                                }
                                }
                                }
                                }
                                frame #4 {
                                n467 = VISA Close(VISA resource name=w592, error in (no error)=w591) -> (error out=→"错误输出 2":errorcluster)
                                }
                                frame #5 {
                                # "可视化"
                                # "数据采集"
                                n468 = property on="当前设定温度℃" class="DigNum (严格)"() -> ("Value"=w599:dbl)  [unwired: 2 in, 2 out]
                                n469 = property on="GWS" class="VISAName"() -> (error out=w598:errorcluster, "Value"=w597:refnum<visa-resource-name>)  [unwired: 2 in, 1 out]
                                n470 = while {
                                tunnel: w597 -> [w604]
                                tunnel: w598 -> [w603]
                                tunnel: w599 -> [w602]
                                tunnel: [w601] -> w596
                                tunnel: [w600] -> w593
                                stop <- w601 stop-if-true
                                w605 = 0.1
                                # "再次判断温度设置"
                                n471 = call "get_temp.vi"("错误输入（无错误）"=w603, "VISA资源名称"=w604) -> ("实时温度"=w600:dbl)  [unwired: 7 in, 2 out]
                                n472 = property on="实时温度℃" class="DigNum (严格)"("Value"=w600) -> ()  [unwired: 2 in, 2 out]
                                n473 = Add(x=w602, y=w605) -> (x+y=w606:dbl)
                                n474 = Subtract(x=w602, y=w605) -> (x-y=w607:dbl)
                                n475 = In Range and Coerce(upper limit=w606, x=w600, lower limit=w607) -> (In Range?=w601:bool)  [unwired: 1 out]
                                }
                                n476 = And(x=w595, y=w596) -> (x .and. y?=w594:bool)
                                n477 = case shown="真" w594 {
                                tunnel: w593 -> [_ w609]
                                frame False {
                                }
                                frame True {
                                w612 = u16 0 items=["DC Voltage", "AC Voltage", "2 - Wire Resistance", "4 - Wire Resistance", "DC Current", "AC Current", "Frequency", "Period", "Continuity", "Diode Checking", "VDC:VDC Ratio", "Temperature", "Capacitance"] ("Function (0: DC Voltage)")
                                w620 = ""
                                n478 = property on="传感器顺序编号（从1开始）" class="Arr (严格)"() -> ("Value"=w623:string[])  [unwired: 2 in, 2 out]
                                n479 = property on="HP34401" class="VISAName"() -> ("Value"=w613:refnum<visa-resource-name>)  [unwired: 2 in, 2 out]
                                n480 = Get Date/Time String(want seconds? (F)=TRUE ("disable buffering (T)")) -> (time string=w632:string)  [unwired: 2 in, 1 out]
                                n481 = property on="实时压力kPa" class="Str"() -> ("Value"=w630:string)  [unwired: 2 in, 2 out]
                                n482 = Number To Fractional String(number=w609) -> (F-format string=w631:string)  [unwired: 3 in]
                                n483 = Array Size(array=w623) -> (size(s)=w629:i32)
                                n484 = Interleave 1D Arrays(w623, string[] [" ", " ", " ", " ", " ", " ", " ", " ", " ", " "]) -> (w621:string[])
                                n485 = Multiply(x=2, y=w629) -> (x*y=w611:i32)
                                n486 = for {
                                N: w611 -> [_]
                                tunnel: w613 -> [w637]
                                tunnel: w612 -> [w636]
                                tunnel: [w634] -> w610 mode=indexing
                                n487 = call "Agilent 34401.vi"("Function (0: DC Voltage)"=w636, "VISA resource name"=w637) -> ("Measurement"=w635:dbl)  [unwired: 1 in, 1 out]
                                n488 = Number To Fractional String(number=w635) -> (F-format string=w634:string)  [unwired: 3 in]
                                }
                                n489 = Add(x=3, y=w611) -> (x+y=w624:i32)
                                n490 = property on="数据" class="Arr (严格)"() -> ("Value"=w617:string[][])  [unwired: 2 in, 2 out]
                                n491 = Build Array (concatenate)(w632, w631, w630, w610) -> (w616:string[])
                                n492 = Build Array (concatenate)(w620, w620, w620, w621) -> (w618:string[])
                                n493 = Array Subset(array=string[] ["时间", "温度（℃）", "压力（KPa）", "电压1（V）", "桥压1（V）", "电压2（V）", "桥压2（V）", "电压3（V）", "桥压3（V）", "电压4（V）", "桥压4（V）", "电压5（V）", "桥压5（V）"], index=0 ("索引"), length=w624) -> (w619:string[])
                                n494 = Build Array (concatenate)(w617, w616) -> (w614:string[][])
                                n495 = Build Array(w619, w618) -> (w615:string[][])
                                n496 = Insert Into Array(array=w615, new element=w614) -> (w608:string[][])  [unwired: 2 in]
                                n497 = property on="数据" class="Arr (严格)"("Value"=w614) -> ()  [unwired: 2 in, 2 out]
                                n498 = property on="显示数据" class="MCListbox (严格)"("ItemNames"=w608) -> ()  [unwired: 2 in, 2 out]
                                }
                                }
                                }
                                frame #6 {
                                n499 = property on="压力稳定" class="Bool (严格)"("Value"=FALSE ("压力稳定")) -> ()  [unwired: 2 in, 2 out]
                                }
                                }
                                }
                              }
                              frame #1 {
                                n500 = property on="开始采集" class="Bool (严格)"("Value"=FALSE ("开始采集")) -> ()  [unwired: 2 in, 2 out]
                                n501 = property on="压力稳定" class="Bool (严格)"("Value"=FALSE ("压力稳定")) -> ()  [unwired: 2 in, 2 out]
                                n502 = property on="结束" class="Bool (严格)"("Value"=TRUE ("结束")) -> ()  [unwired: 2 in, 2 out]
                              }
                            }
                          }
                        }
                      }
                    }
                  }
                  frame #6 {
                    # "关闭"
                    n503 = property on="结束" class="Bool (严格)"() -> ("Value"=w761:bool)  [unwired: 2 in, 2 out]
                    n504 = case shown="真" w761 {
                      frame False {
                      }
                      frame True {
                        w790 = "Measured Data"  # group name
                        w789 = string[] ["时间", "温度", "压力", "电压1", "桥压1（V）", "电压2", "桥压2", "电压3", "桥压3", "电压4", "桥压4", "电压5", "桥压5"]  # channel names
                        # "恢复压力到常压"
                        # "结束"
                        # "数据保存"
                        n505 = property on="温度（℃）" class="Arr (严格)"() -> ("Value"=w788:dbl[])  [unwired: 2 in, 2 out]
                        n506 = property on="温度点" class="DigNum (严格)"() -> ("Value"=w787:i32)  [unwired: 2 in, 2 out]
                        n507 = property on="当前设定温度℃" class="DigNum (严格)"() -> ("Value"=w774:dbl)  [unwired: 2 in, 2 out]
                        n508 = property on="loging" class="Str"() -> ("Value"=w785:string)  [unwired: 2 in, 2 out]
                        n509 = Increment(x=w787) -> (x+1=w809:i32)
                        n510 = Index Array(array=w788, index=w787) -> ()  [unwired: 1 out]
                        n511 = Array Size(array=w788) -> (size(s)=w810:i32)
                        n512 = property on="温度校验次数" class="DigNum (严格)"("Value"=1.0 ("温度校验次数")) -> ()  [unwired: 2 in, 2 out]
                        n513 = Number To Fractional String(number=w774, precision (6)=i16 1 ("精度(6)")) -> (F-format string=w784:string)  [unwired: 2 in]
                        n514 = Concatenate Strings(w785, w784, "℃ " ("字符串"), "数据保存" ("字符串"), "\n") -> (w782:string)
                        n515 = property on="loging" class="Str"("Value"=w782) -> ()  [unwired: 2 in, 2 out]
                        n516 = Equal?(x=w809, y=w810) -> (x = y?=w778:bool)
                        n517 = case shown="真" w778 {
                          tunnel: w809 -> [w833 _]
                          tunnel: [w833 0] -> w808
                          frame False {
                          }
                          frame True {
                            w840 = u16 10 items=["1.0"=10, "1.5"=15, "2.0"=20] ("Serial Settings:Stop Bits")
                            w841 = u16 0 items=["None", "Odd", "Even", "Mark", "Space"] ("Serial Settings:Parity")
                            w839 = "\u000200014000.0000"
                            # "关闭电源"
                            n518 = property on="GWS" class="VISAName"() -> ("Value"=w855:refnum<visa-resource-name>)  [unwired: 2 in, 2 out]
                            n519 = property on="DH1766-2" class="VISAName"() -> ("Value"=w845:refnum<visa-resource-name>)  [unwired: 2 in, 2 out]
                            n520 = call "CRC.vi"("命令字符串"=w839) -> ("校验字符串"=w846:string)  [unwired: 10 in]
                            n521 = Concatenate Strings(w839, w846, "\u0003" ("字符串")) -> (w849:string)
                            n522 = property class="Instr"(reference=w855, "Baud"=u32 19200 ("Serial Settings:Baud Rate"), "Data Bits"=u16 8 ("Serial Settings:Data Bits"), "Parity"=w841, "Stop Bits"=w840) -> (reference out=w852:refnum<visa-resource-name>)  [unwired: 1 in, 1 out]
                            n523 = call-poly "VISA Configure Serial Port"("VISA resource name"=w845, "Enable Termination\nChar (T)"=FALSE ("Enable Termination\nChar (T)"), "baud rate (9600)"=u32 9600) -> ("VISA resource name out"=w850:refnum<visa-resource-name>, "error out"=w851:errorcluster)  [unwired: 4 in, 7 out]
                            n524 = property on="START" class="Bool (严格)"("Value"=FALSE ("START")) -> ()  [unwired: 2 in, 2 out]
                            n525 = VISA Write(VISA resource name=w850, write buffer=w849, error in (no error)=w851) -> (VISA resource name out=w847:refnum<visa-resource-name>, error out=w848:errorcluster)  [unwired: 1 out]
                            n526 = VISA Write(VISA resource name=w852, write buffer="MODE,OFF" ("写入缓冲区")) -> (VISA resource name out=w854:refnum<visa-resource-name>, error out=w853:errorcluster)  [unwired: 1 in, 1 out]
                            n527 = VISA Close(VISA resource name=w847, error in (no error)=w848) -> ()  [unwired: 1 out]
                            n528 = property on="时漂测试" class="Bool (严格)"("Value"=FALSE ("时漂测试")) -> ()  [unwired: 2 in, 2 out]
                            n529 = VISA Close(VISA resource name=w854, error in (no error)=w853) -> ()  [unwired: 1 out]
                          }
                        }
                        n530 = property on="温度点" class="DigNum (严格)"("Value"=w808) -> ()  [unwired: 2 in, 2 out]
                        n531 = property on="结束" class="Bool (严格)"("Value"=FALSE ("结束")) -> ()  [unwired: 2 in, 2 out]
                        n532 = property on="时漂测试" class="Bool (严格)"() -> ("Value"=w776:bool)  [unwired: 2 in, 2 out]
                        n533 = property on="GWS" class="Bool (严格)"("Value"=FALSE ("GWS")) -> ()  [unwired: 2 in, 2 out]
                        n534 = case shown="真" w776 {
                          tunnel: [w830 w832] -> w777
                          frame False {
                            n535 = property on="数据" class="Arr (严格)"() -> ("Value"=w830:string[][])  [unwired: 2 in, 2 out]
                          }
                          frame True {
                            n536 = property on="时漂常压输出" class="Arr (严格)"() -> ("Value"=w832:string[][])  [unwired: 2 in, 2 out]
                            n537 = property on="时漂测试" class="Bool (严格)"("Value"=FALSE ("时漂测试")) -> ()  [unwired: 2 in, 2 out]
                          }
                        }
                        n538 = Transpose 2D Array(2D array=w777) -> (transposed array=w797:string[][])
                        n539 = Current VI's Path() -> (path=w775:path)
                        n540 = Strip Path(path=w775) -> (stripped path=w801:path)  [unwired: 1 out]
                        n541 = property on="数据保存路径" class="Path"() -> ("Value"=w796:path)  [unwired: 2 in, 2 out]
                        n542 = disable-structure shown="禁用" {
                          frame Disabled {
                            # "不同温度下的满量程输出值"
                            n543 = property on="压力设定值（KPa）" class="Arr (严格)"() -> ("Value"=w818:dbl[])  [unwired: 2 in, 2 out]
                            n544 = Array Max & Min(array=w818) -> (max value=w817:dbl)  [unwired: 3 out]
                            n545 = Divide(x=w817, y=1000.0) -> (x/y=w816:dbl)
                            n546 = Multiply(x=w816) -> (y=w819:dbl, x*y=→"Yf.s":dbl)
                          }
                          frame Enabled {
                          }
                        }
                        n547 = Build Path(base path=w801, name or relative path="data" ("字符串")) -> (appended path=w800:path)
                        n548 = property on="检定次数" class="DigNum (严格)"() -> ("Value"=w772:i32)  [unwired: 2 in, 2 out]
                        n549 = property on="压力设定值（KPa）" class="Arr (严格)"() -> ("Value"=w773:dbl[])  [unwired: 2 in, 2 out]
                        n550 = Build Path(base path=w800, name or relative path=w796) -> (appended path=w804:path)
                        n551 = Array Size(array=w773) -> (size(s)=w771:i32)
                        n552 = property on="传感器显示编号" class="Enum (严格)"() -> ("Value"=w768:enum16{""})  [unwired: 2 in, 2 out]
                        n553 = case shown="真" w776 {
                          tunnel: [w820 w822] -> w769
                          tunnel: w768 -> [_ w823]
                          frame False {
                            n554 = property on="数据" class="Arr (严格)"() -> ("Value"=w820:string[][])  [unwired: 2 in, 2 out]
                          }
                          frame True {
                            n555 = disable-structure shown="禁用" {
                              frame Disabled {
                                n556 = property on="温度（℃）" class="Arr (严格)"() -> ("Value"=w828:dbl[])  [unwired: 2 in, 2 out]
                                n557 = call "getNormalTempIndex.vi"("温度列表"=w828) -> ("常温索引"=w829:dbl)  [unwired: 10 in]
                                n558 = Index Array(index=w829) -> ()  [unwired: 1 in, 1 out]
                              }
                              frame Enabled {
                              }
                            }
                            n559 = property on="时漂常压输出" class="Arr (严格)"() -> ("Value"=w826:string[][])  [unwired: 2 in, 2 out]
                            n560 = call "getTimeMov.vi"("Yf·s"=4.6, "传感器索引"=w823, "不包含头的全量数组数据"=w826) -> ("时漂"=→"时漂":dbl)  [unwired: 8 in]
                            n561 = call "getDataFromTDMS.vi"("文件名称"="test") -> ("数据"=w822:string[][])  [unwired: 10 in]
                            n562 = property on="时漂测试" class="Bool (严格)"("Value"=FALSE ("时漂测试")) -> ()  [unwired: 2 in, 2 out]
                          }
                        }
                        n563 = TDMS Open(6:FALSE ("disable buffering (T)"), 7:enum16{"1.0", "2.0"}."2.0" ("file format version (2.0)"), 10:T3."open or create" ("operation"), 11:w804) -> (0:w802:errorcluster, 3:w799:refnum<k34>)  [unwired: 3 in]
                        n564 = call "getCluster.vi"("数据"=w769, "检定次数"=w772, "压力点个数"=w771, "传感器索引（1开始）"=w768) -> ("结果簇"=→"XY图":cluster{dbl[], dbl[]}[], "曲线信息"=w766:string[])  [unwired: 4 in, 6 out]
                        n565 = property on="CONST820" class="VISAName"() -> ("Value"=w780:refnum<visa-resource-name>)  [unwired: 2 in, 2 out]
                        n566 = call "setConst820.vi"("VISA resource name"=w780, "输入命令"="output:MODE VENT") -> ("VISA资源名称输出"=w763:refnum<visa-resource-name>, "错误输出"=w762:errorcluster)  [unwired: 6 in, 1 out]
                        n567 = TDMS Write(0:w799, 1:enum16{"decimated", "interleaved"}."decimated" ("数据布局（0:降采样）"), 5:w790, 7:w789, 9:w797, 11:w802) -> (4:w798:refnum<k34>, 15:w803:errorcluster)  [unwired: 2 out]
                        n568 = for {
                          tunnel: w766 -> [w811] mode=indexing
                          shift-right: [w813] -> w764
                          shift-left: "" -> [w812]
                          n569 = Concatenate Strings(w812, w811) -> (w813:string)
                        }
                        n570 = TDMS Close(8:w803, 11:w798) -> ()  [unwired: 2 out]
                        n571 = VISA Close(VISA resource name=w763, error in (no error)=w762) -> ()  [unwired: 1 out]
                        n572 = property on="曲线拟合参数" class="Str"("Value"=w764) -> ()  [unwired: 2 in, 2 out]
                      }
                    }
                  }
                }
              }
              frame True {
                n573 = call "显示对话框信息"("Message"=w857) -> ()  [unwired: 9 in, 2 out]
                n574 = property on="START" class="Bool (严格)"("Value"=FALSE ("START")) -> ()  [unwired: 2 in, 2 out]
              }
            }
          }
        }
      }
    }
  }
